vi "FGV_Instrument_Class.vi"(0 "Action":T2(ring), 5 "Instruments":T1(array[cluster]), 7 "Instr class":string, 9 "Instr name":string, 11 "error in (no error)":errorcluster, 12 "Parameter":string, 13 "Familly class IN":refnum<class "Class Instrument (Default).lvclass">) -> (4 "Instruments 2":T1(array[cluster]), 6 "Familly class Out":refnum<class "Class Instrument (Default).lvclass">, 15 "error out":errorcluster)   [LabVIEW 2020, in "Library Commun.lvlib"]
uses:
  Library Commun.lvlib
  Class/Instrument/Instrument (Default)/Class Instrument (Default).lvclass
  Class/Instrument/Instrument Firebase Altyor/Class Instrument Firebase Altyor.lvclass
  C:/Users/ngarcin/OneDrive - Altyor/Standard TB/Class/Instrument/Instrument (Default)/Class Instrument (Default).lvclass
  Class/Firebase/Source/Firebase Altyor/Firebase Altyor.lvclass
  Class/DIO/Class DIO NI/Class DIO NI.lvclass
  C:/Users/ngarcin/OneDrive - Altyor/Standard TB/Class/DIO/Class DIO (Default)/Class DIO (Default).lvclass
  TypeDef/Commande DIO/Parameter DIO.ctl
  Class/DIO/Class DIO (Default)/Class DIO (Default).lvclass
  Class/Instrument/Instrument DIO/Class Instrument DIO.lvclass
  Class/Ana/Class Ana NI/Class Ana NI.lvclass
  C:/Users/ngarcin/OneDrive - Altyor/Standard TB/Class/Ana/Class Ana (Default)/Class Ana (Default).lvclass
  Class/Ana/Class Ana (Default)/Class Ana (Default).lvclass
  Class/Instrument/Instrument Ana/Class Instrument Ana.lvclass
  Class/Multimeter/Multimeter Rigol DM3058/Class Multimeter Rigol DM3058.lvclass
  C:/Users/ngarcin/OneDrive - Altyor/Standard TB/Class/Multimeter/Multimeter (Default)/Class Multimeter (Default).lvclass
  Class/Multimeter/Multimeter (Default)/Class Multimeter (Default).lvclass
  TypeDef/Command Multimeter/Parameter Multimeter.ctl
  TypeDef/Command Multimeter/Typedef Function.ctl
  Class/Instrument/Class Instrument Multimeter/Class Instrument Multimeter.lvclass
  Class/Power_Supply/Power_Supply Rigol DP832/Class Power_Supply Rigol DP800.lvclass
  C:/Users/ngarcin/OneDrive - Altyor/Standard TB/Class/Power_Supply/Power_Supply (Default)/Power_Supply (Default).lvclass
  Class/Instrument/Instrument Power_Supply/Class Instrument Power_Supply.lvclass
  Class/Power_Supply/Power_Supply (Default)/Power_Supply (Default).lvclass
  TypeDef/Command Power_Supply/Parameter Power_Supply.ctl
  Class/Relay_Board/Relay_Board 16_Relay_Acer_Micro/Class Relay_Board 16_Relay_Acer_Micro.lvclass
  Class/Relay_Board/Relay_Board (Default)/Class Relay_Board (Default).lvclass
  Class/Instrument/Instrument Relay_Board/Class Instrument Relay_Board.lvclass
  Class/Relay_Board/Class Relay_Board 16_Relay_R4D3B16/Class Relay_Board 16_Relay_R4D3B16.lvclass
  C:/Users/ngarcin/OneDrive - Altyor/Standard TB/Class/Relay_Board/Relay_Board (Default)/Class Relay_Board (Default).lvclass
  TypeDef/Commande Relay_Board/Parameter Relay_Board.ctl
  Class/Relay_Board/Class Relay_Board 8_Relay_N4D8B08/Class Relay_Board 8_Relay_N4D8B08.lvclass
  Class/Relay_Board/Class Relay_Board 8_Relay_RY408D/Class Relay_Board 8_Relay_RY408D.lvclass
  Class/Relay_Board/Relay_Board usb_Relay_device/Class Relay_Board usb_Relay_device.lvclass
  TypeDef/Commande Printer/Commande Parameter Printer.ctl
  Class/Printer/Printer (Default)/Class Printer (Default).lvclass
  Class/Instrument/Instrument Printer/Class Instrument Printer.lvclass
  Class/Printer/Printer CAB/Class Printer_CAB.lvclass
  C:/Users/ngarcin/OneDrive - Altyor/Standard TB/Class/Printer/Printer (Default)/Class Printer (Default).lvclass
  Class/Printer/Printer TSC/Class Printer_TSC.lvclass
  Class/Instrument/Instrument Schielding_Box/Class Instrument Schielding_Box.lvclass
  Class/Shielding box/Class Shielding_ Box JC-PB3044/Class Shielding_ Box JC-PB3044.lvclass
  C:/Users/ngarcin/OneDrive - Altyor/Standard TB/Class/Shielding box/Class Shielding box (Default)/Class Shielding_ Box (Default).lvclass
  Class/Shielding box/Class Shielding box (Default)/Class Shielding_ Box (Default).lvclass
  TypeDef/Commande Shielding box/Commande Shielding box.ctl
  Class/Spectrum Analyser/Class Spectrum_Analyser RS306B/Class Spectrum_Analyser RS306B.lvclass
  C:/Users/ngarcin/OneDrive - Altyor/Standard TB/Class/Spectrum Analyser/Class Spectrum Analyser (Default)/Class Spectrum Analyser (Default).lvclass
  Class/Spectrum Analyser/Class Spectrum Analyser (Default)/Class Spectrum Analyser (Default).lvclass
  TypeDef/Command Spectrum_Analyser/Parameter Spectrum_Analyser.ctl
  Class/Instrument/Instrument Spectrum_Analyser/Class Instrument Spectrum_Analyser.lvclass
  TypeDef/Commande Led_Analyser/Parametre LED analyser.ctl
  Class/LED Analyser/Class Led Analyser (Default)/Class LED Analyser (Default).lvclass
  Class/LED Analyser/FEASA/LED Analyser FEASA_10_F/Class LED Analyser FEASA_10_F.lvclass
  C:/Users/ngarcin/OneDrive - Altyor/Standard TB/Class/LED Analyser/Class Led Analyser (Default)/Class LED Analyser (Default).lvclass
  Class/Instrument/Instrument LED_Analyser/Class Instrument LED_Analyser.lvclass
  TypeDef/Command firebase altyor/Parameter Firebase Altyor.ctl
  TypeDef/Bench Type.ctl
  Class/Firebase/Source/Firebase AssembledProducts/Firebase AssembledProducts.lvclass
  C:/Users/ngarcin/OneDrive - Altyor/Standard TB/Class/Firebase/Source/Firebase Altyor/Firebase Altyor.lvclass
  Class/Instrument/Instrument Database Altyor/Class Instrument Database Altyor.lvclass
  Class/Database/Database Altyor/Database Altyor.lvclass
  Class/Firebase/Source/Firebase PCBA/Firebase Benches.lvclass
  Class/Instrument/Instrument UART/Class Instrument UART.lvclass
  Class/UART/UART Enocean/Class UART Enocean.lvclass
  C:/Users/ngarcin/OneDrive - Altyor/Standard TB/Class/UART/UART (Default)/Class UART (Default).lvclass
  TypeDef/Commande UART/Parametre UART.ctl
  Class/UART/UART (Default)/Class UART (Default).lvclass
  Class/UART/UART Nodon/Class UART Nodon.lvclass
  Class/UART/UART P2056/Class UART P2056/Class UART P2056.lvclass
  Class/UART/UART Zigbee/Class UART Zigbee.lvclass
  Class/Camera/Class Camera IV3-500CA (Default)/Class Camera IV3-500CA.lvclass
  C:/Users/ngarcin/OneDrive - Altyor/Standard TB/Class/Camera/Class Camera Pattern Matching (Default)/Class Pattern Matching (Default).lvclass
  Class/Instrument/Instrument Pattern_Matching/Class Instrument Patterm_Matching.lvclass
  TypeDef/Commande Pattern_Matching/Commande Parameter.ctl
  Class/Camera/Class Camera Pattern Matching (Default)/Class Pattern Matching (Default).lvclass
  Class/Balance/Adam_GBK/Class Balance_Adam_GBK.lvclass
  C:/Users/ngarcin/OneDrive - Altyor/Standard TB/Class/Balance/Balance (Default)/Class Balance (Default).lvclass
  Class/Balance/Balance (Default)/Class Balance (Default).lvclass
  TypeDef/Commande Balance/Parameter Balance.ctl
  Class/Instrument/Instrument Balance/Class Instrument Balance.lvclass
  Class/Instrument/Instrument Log_File/Class Instrument Log_File.lvclass
  TypeDef/Commande Test/Commande Data Test.ctl
  TypeDef/Commande Test/Commande Value Type.ctl
  TypeDef/Commande Test/Commande Type Test.ctl
  Class/Log File/Class Log_File Altyor/Class Log_File Altyor.lvclass
  Class/JSON API/JSON Value/Set from JSON string.vi
  Class/JSON API/Variant JSON/Variant to JSON.vi
  Class/JSON API/JSON Value/Get Item by name array.vi
  Class/JSON API/JSON Value/JSON Value.lvclass
  Class/JSON API/Get Polymorphic/JSON GetSet.lvlib
  Class/JSON API/Variant JSON/Variant JSON.lvlib
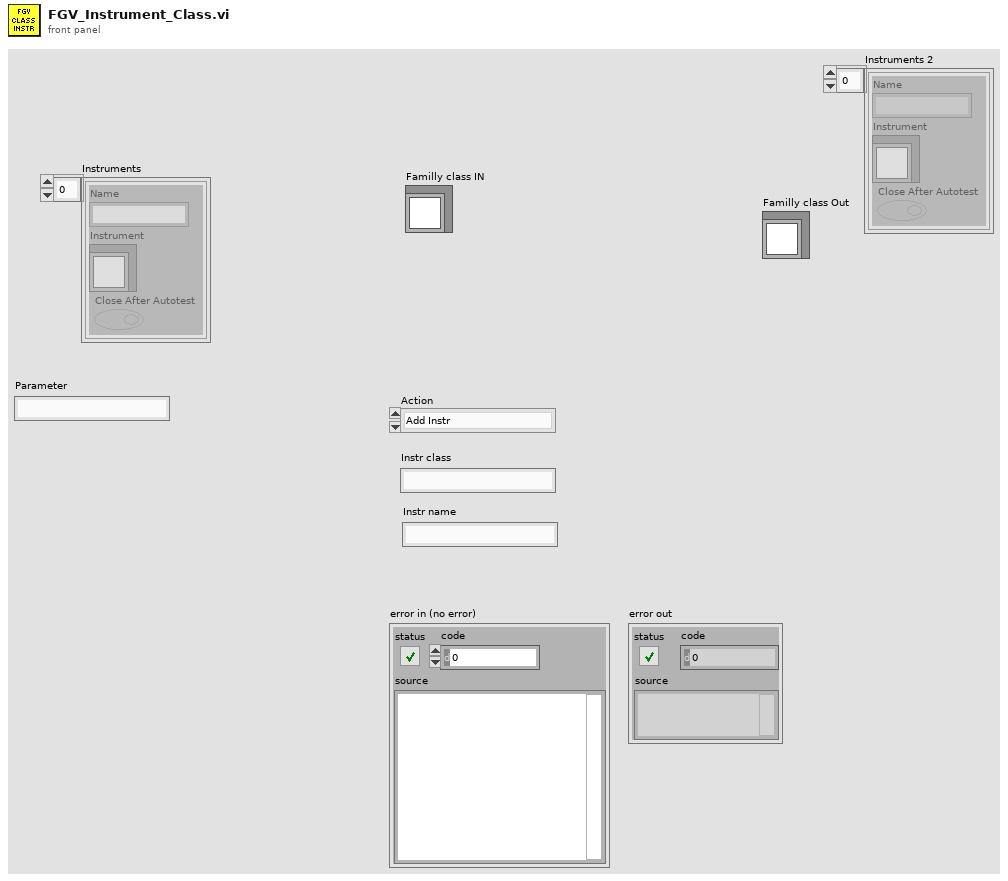
[diagram p1: front panel]
types:
  T1 = cluster{"Name":string, "Instrument":refnum<class "Class Instrument (Default).lvclass">, "Close After Autotest":bool}[]
  T2 = enum16{"Add Instr", "Remove Instr", "List Instr", "Get Instr Class", "Get Instr obj", "Save Insrt obj", "Modify Insrt obj", "Init"}
  T3 = typedef "Parameter DIO.ctl" = cluster{"Device_Com_Port":string, "Port":u8, "Line":u8, "Function":enum16{"Write", "Read"}, "Class DIO":refnum<class "Class DIO (Default).lvclass">}
  T4 = cluster{"Device_Com_Port":string, "Rate":u16, "Nb Sample":u16, "Voltage Max":dbl, "Voltage Min":dbl, "Input terminal Configuration":string, "Channel":u8[], "Continuous":bool, "Nb Data_To_Read":i16, "Class Ana":refnum<class "Class Ana (Default).lvclass">}
  T5 = typedef "Library Commun.lvlib/Parameter Multimeter.ctl" = cluster{"Device @":refnum<visa-resource-name>, "Range":dbl, "Voltage Type":enum16{"AC", "DC"}, "Function":T6, "Class Multimeter":refnum<class "Class Multimeter (Default).lvclass">}
  T6 = typedef "Library Commun.lvlib/Typedef Function.ctl" = enum16{"Voltmeter", "Ammeter", "Continuity", "Ohmmeter", "Frequencymeter"}
  T7 = typedef "Library Commun.lvlib/Parameter Relay_Board.ctl" = cluster{"Device_Com_Port":string, "Address Board":string, "Tab_Num_Relay":u8[], "Parameter Class Relay_Board":refnum<class "Class Relay_Board (Default).lvclass">}
  T8 = typedef "Commande Parameter Printer.ctl" = cluster{"Device_Printer":string, "File To print":path, "Path Picture":path, "Library Printer":refnum<class "Class Printer (Default).lvclass">}
  T9 = typedef "Commande Shielding box.ctl" = cluster{"Device @":string, "Class Shielding_ Box":refnum<class "Class Shielding_ Box (Default).lvclass">}
  T10 = typedef "Parameter Spectrum_Analyser.ctl" = cluster{"Device @":string, "Class Spectrum Analyser":refnum<class "Class Spectrum Analyser (Default).lvclass">, "Center Freq (MHz)":dbl, "Freq Span (MHz)":dbl, "Ref Level (dBm)":dbl, "Threshold (dBm)":dbl, "TimeOut":i16}
  T11 = typedef "Parametre LED analyser.ctl" = cluster{"Device @":string, "Channel":u16, "LED Analyser":refnum<class "Class LED Analyser (Default).lvclass">}
  T12 = typedef "Library Commun.lvlib/Parameter Firebase Altyor.ctl" = cluster{"Name_BDD":string, "API_Key":string, "Nb_to_Read":string, "Value_to_find":string, "Field_Filter":string, "Field_Order":string, "Collection_to_find":string, "Name_Bench":string, "Bench Type":T13, "Type Data ":enum16{"Data Product", "Data Test"}, "Firebase Altyor":refnum<class "Firebase Altyor.lvclass">}
  T13 = typedef "Library Commun.lvlib/Bench Type.ctl" = enum16{"Bench PCBA", "Bench Camera", "Bench Assembly", "Bench PCBA P2193"}
  T14 = cluster{"Connection Name ODBC":string, "DatabaseName":string, "Condition":string, "Type Data ":enum16{"Data Product", "Data Test"}, "Database Altyor":refnum<class "Database Altyor.lvclass">}
  T15 = typedef "Parametre UART.ctl" = cluster{"Address Device":refnum<visa-resource-name>, "Baud Rate":u32, "Data Bit":u16, "stop bits (10: 1 bit)":u16, "parity (0:none)":enum16{"None", "Odd", "Even", "Mark", "Space"}, "flow control (0:none)":u16, "termination char ":u8, "Enable Termination":bool, "Nb Octet to Read":u16, "Class UART":refnum<class "Class UART (Default).lvclass">}
  T16 = typedef "Commande Parameter.ctl" = cluster{"Device_Addr":string, "Port":string, "Number Prog":string, "Test Number":u16, "Timeout":u16, "Library Pattern Matching":refnum<class "Class Pattern Matching (Default).lvclass">}
  T17 = typedef "Parameter Balance.ctl" = cluster{"Device @":string, "Timeout":u32, "Class Balance":refnum<class "Class Balance (Default).lvclass">}
  T18 = cluster{"Path_Log_File":path, "Delimit":string, "File For Save":refnum<queue>, "Event Error":refnum<user-event>, "Class Log_File":refnum<class "Class Log_File Altyor.lvclass">}
  T19 = typedef "Library Commun.lvlib/Parameter Power_Supply.ctl" = cluster{"Device_Addr":refnum<visa-resource-name>, "Current":dbl, "Channel":i32, "Voltage":dbl, " Class Power_Supply":refnum<class "Power_Supply (Default).lvclass">}
  T20 = cluster{"Device_Com_Port":string, "Address Board":string}
  T21 = cluster{"Name_BDD":string, "API_Key":string, "Bench Type":T13}
  T22 = cluster{"Connection Name ODBC":string, "DatabaseName":string}
  T23 = cluster{"Address Device":refnum<visa-resource-name>, "Baud Rate":u32, "Data Bit":u16, "stop bits (10: 1 bit)":u16, "parity (0:none)":enum16{"None", "Odd", "Even", "Mark", "Space"}, "flow control (0:none)":u16, "termination char ":u8, "Enable Termination":bool}
  T24 = cluster{"Name":string, "Instrument":refnum<class "Class Instrument (Default).lvclass">, "Close After Autotest":bool}
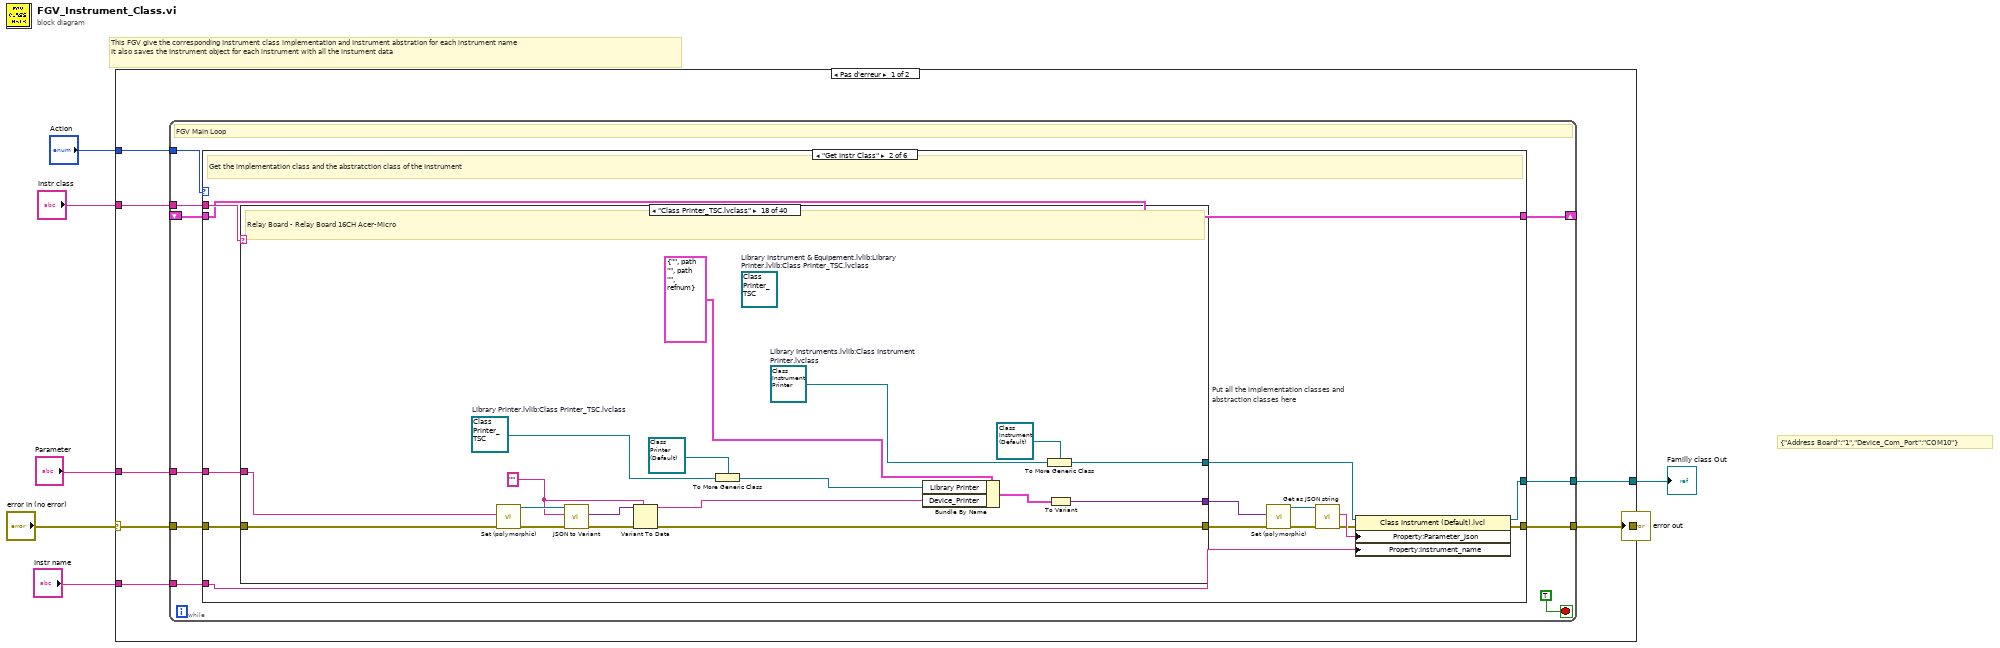
[diagram p0: block diagram]
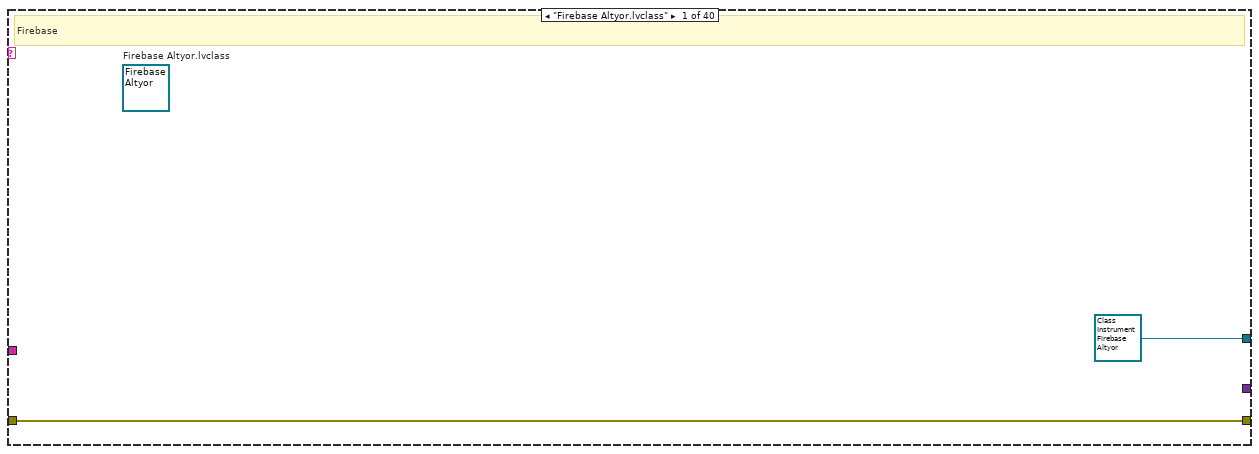
[diagram p3: hidden frame]
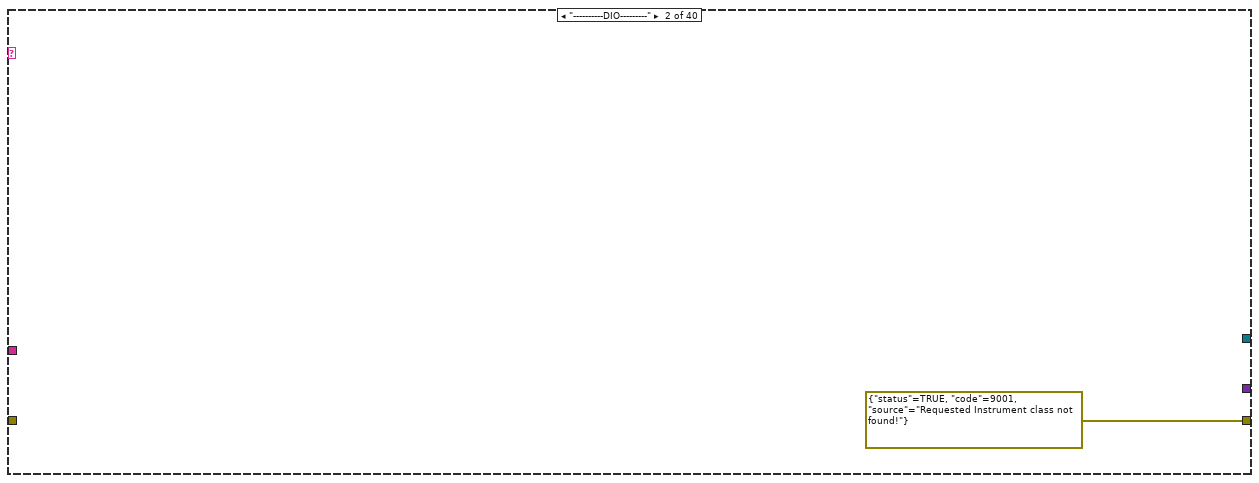
[diagram p4: hidden frame]
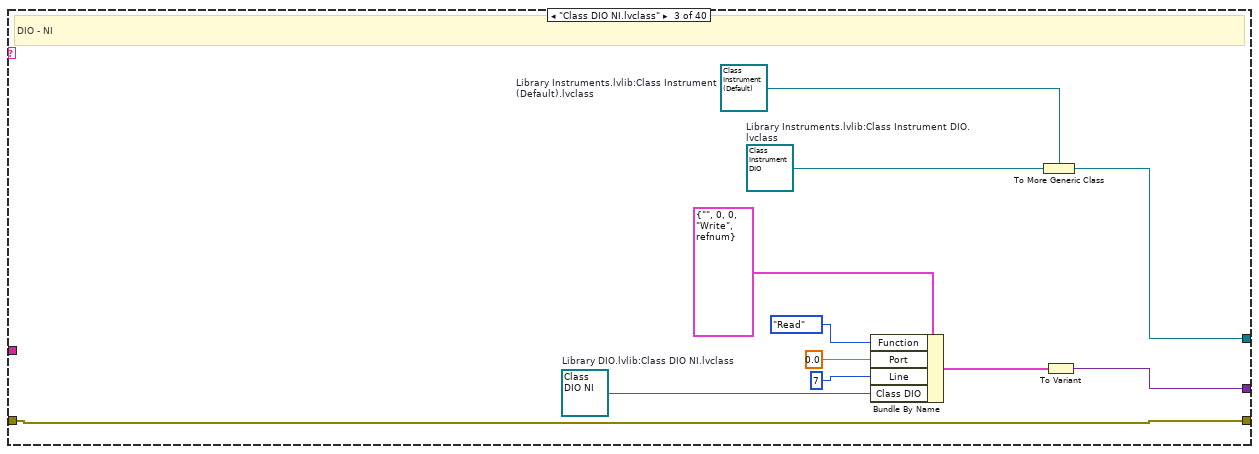
[diagram p5: hidden frame]
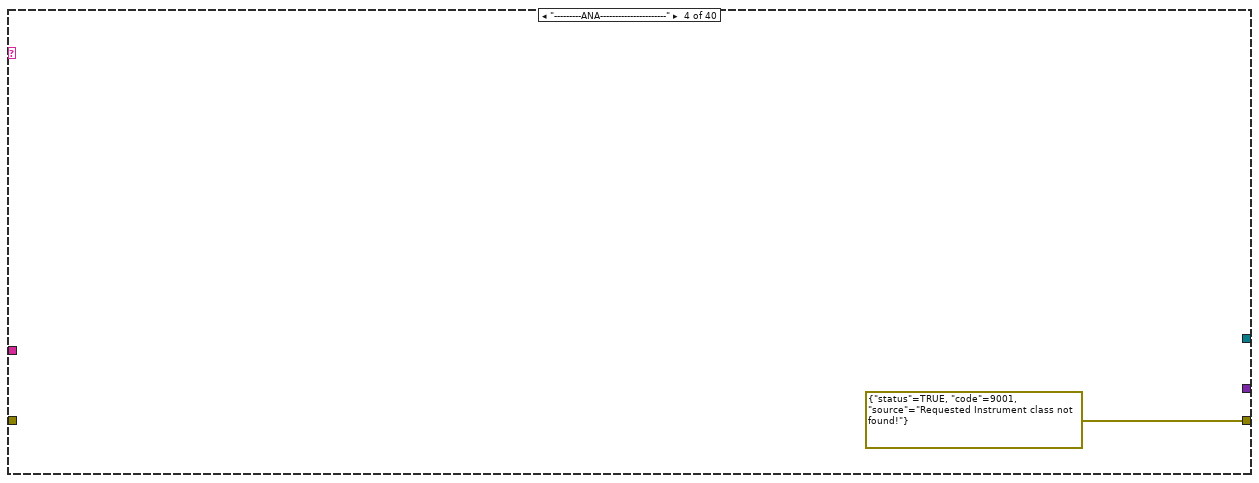
[diagram p6: hidden frame]
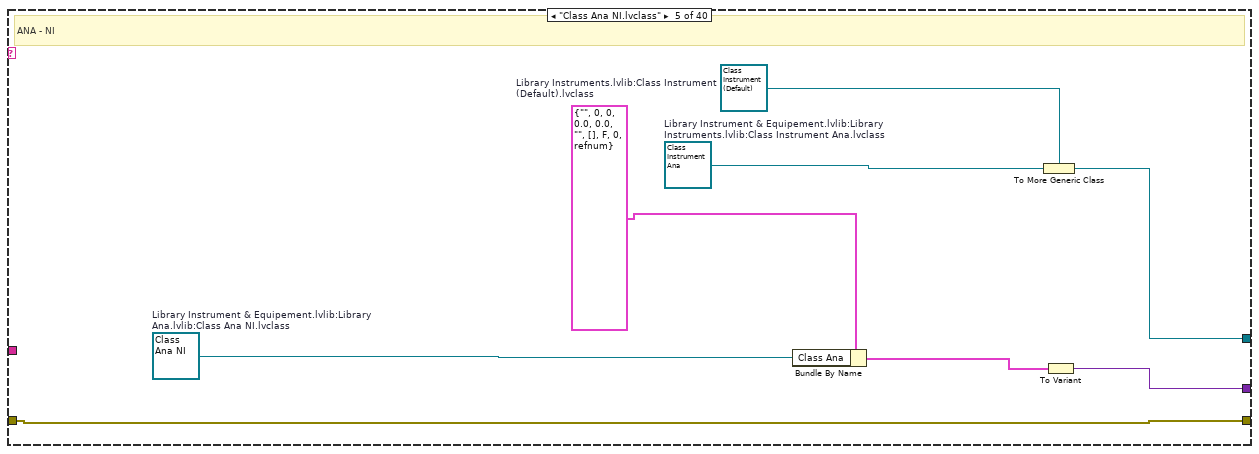
[diagram p7: hidden frame]
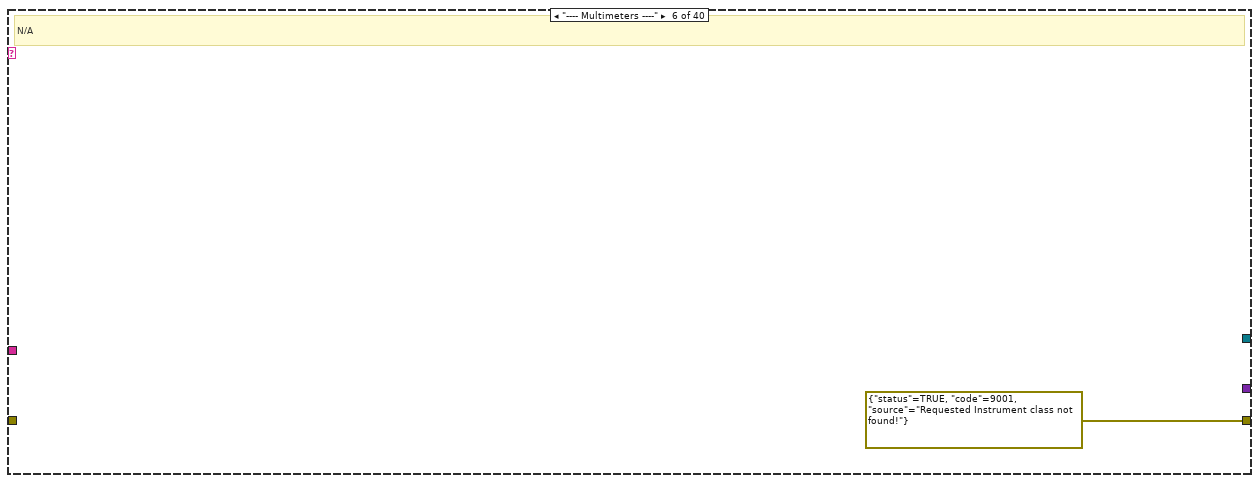
[diagram p8: hidden frame]
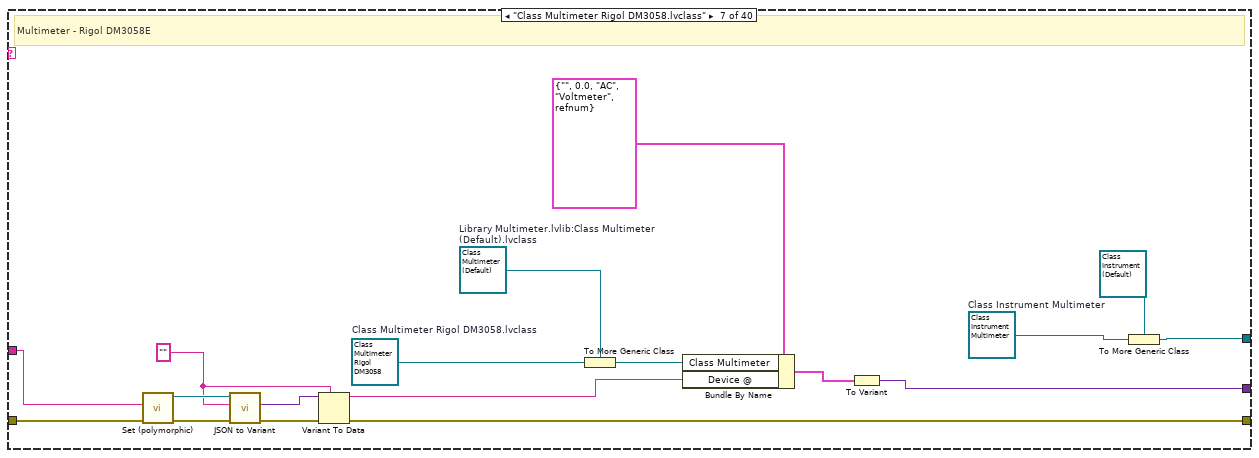
[diagram p9: hidden frame]
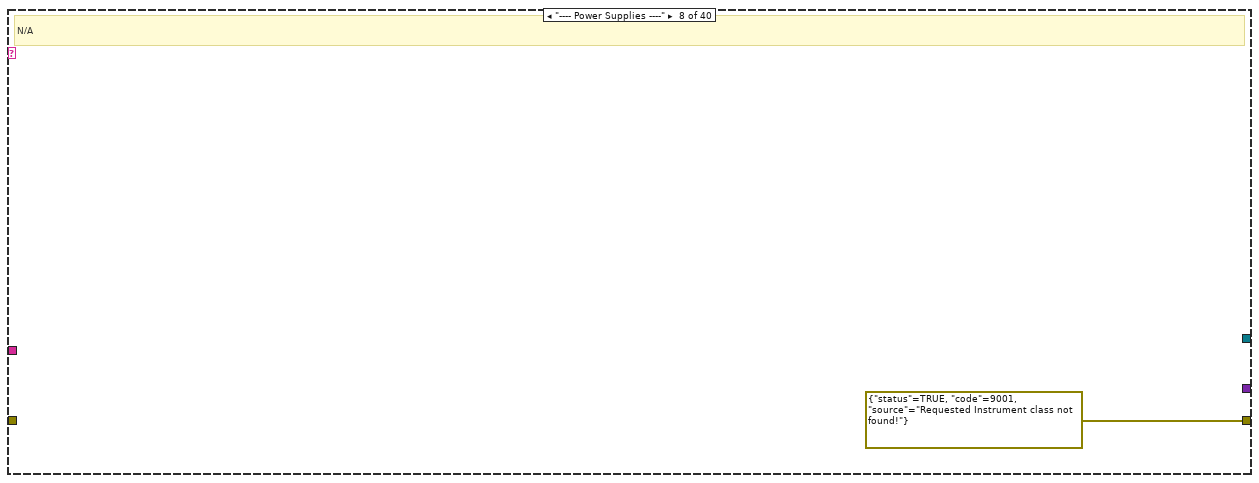
[diagram p10: hidden frame]
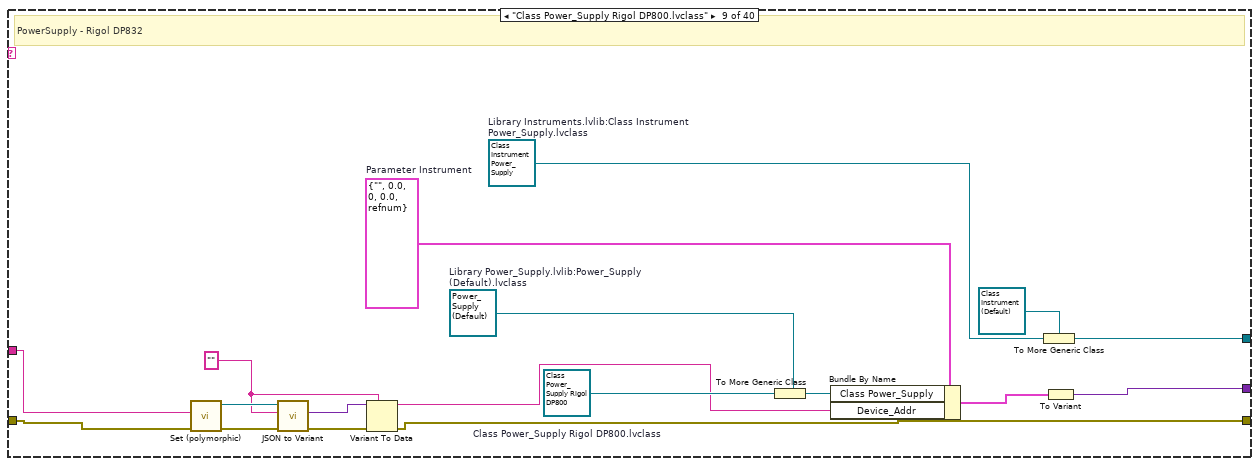
[diagram p11: hidden frame]
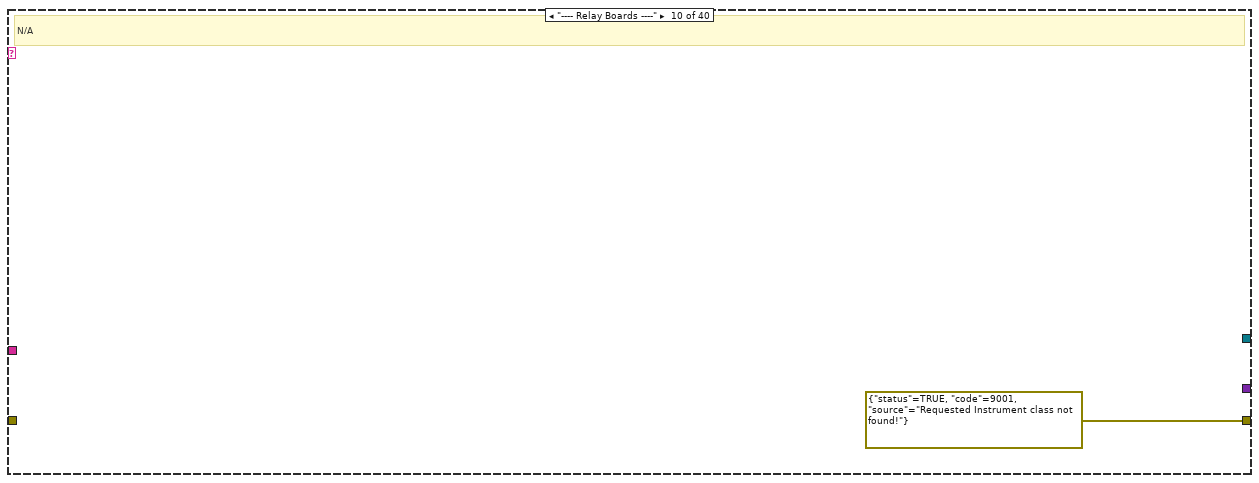
[diagram p12: hidden frame]
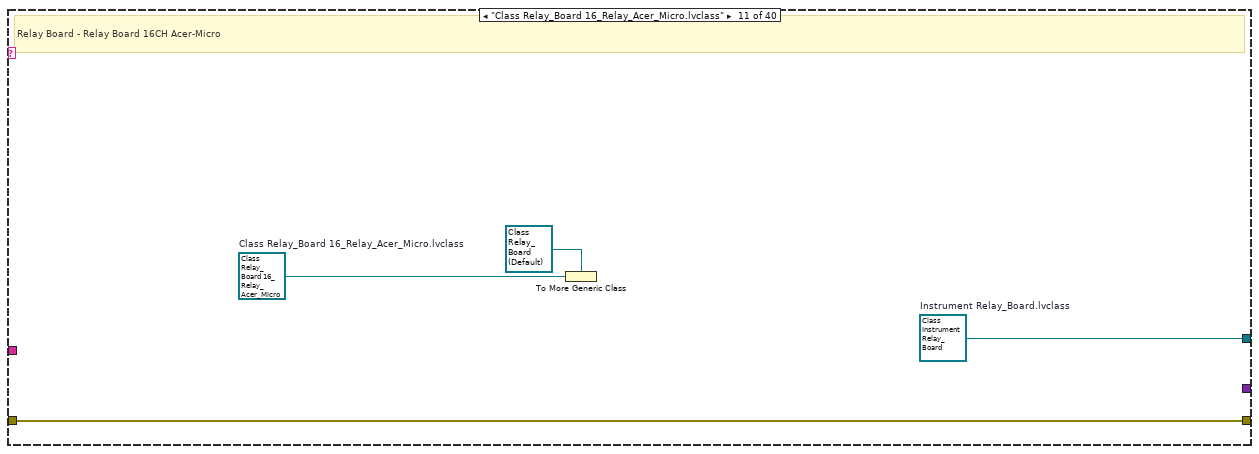
[diagram p13: hidden frame]
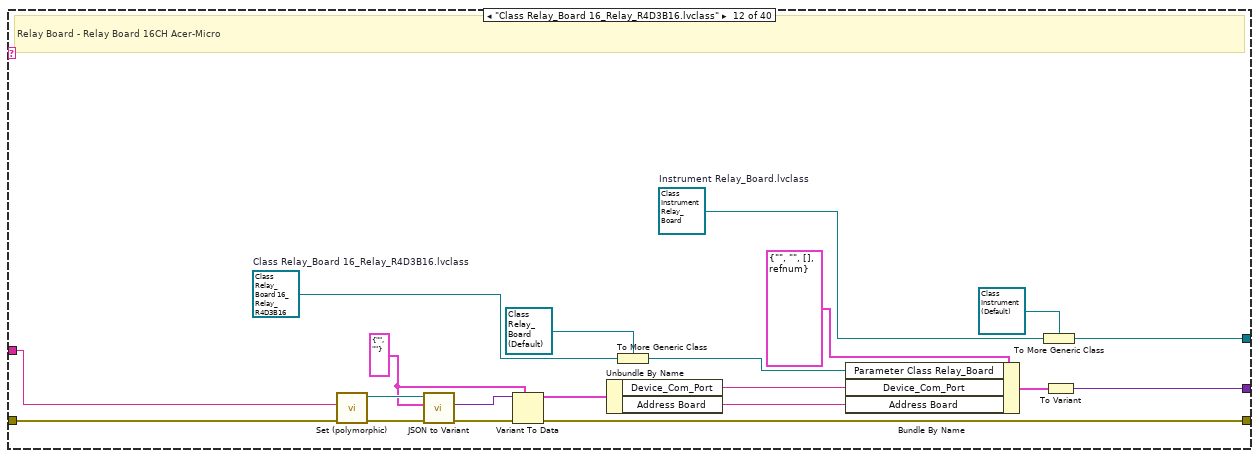
[diagram p14: hidden frame]
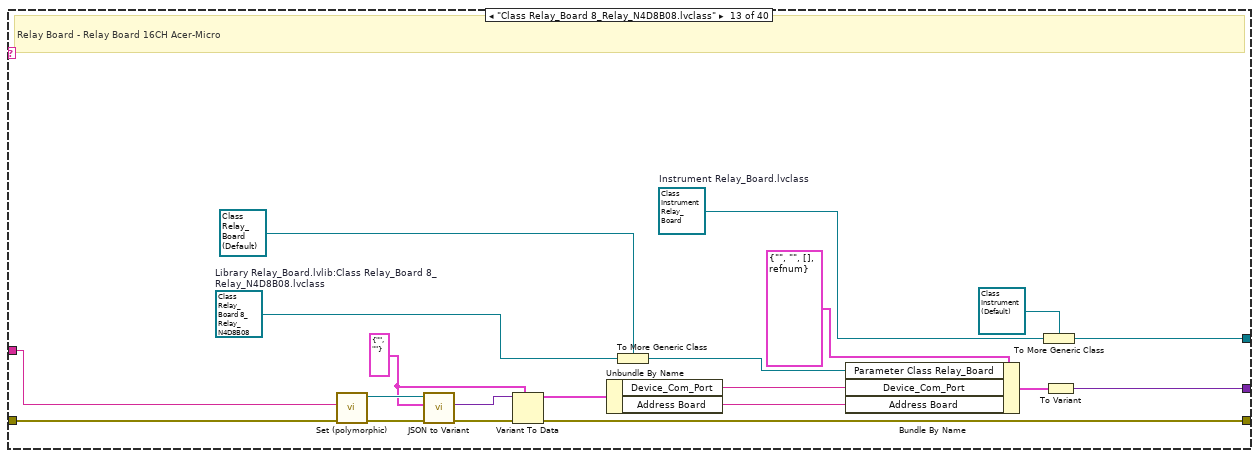
[diagram p15: hidden frame]
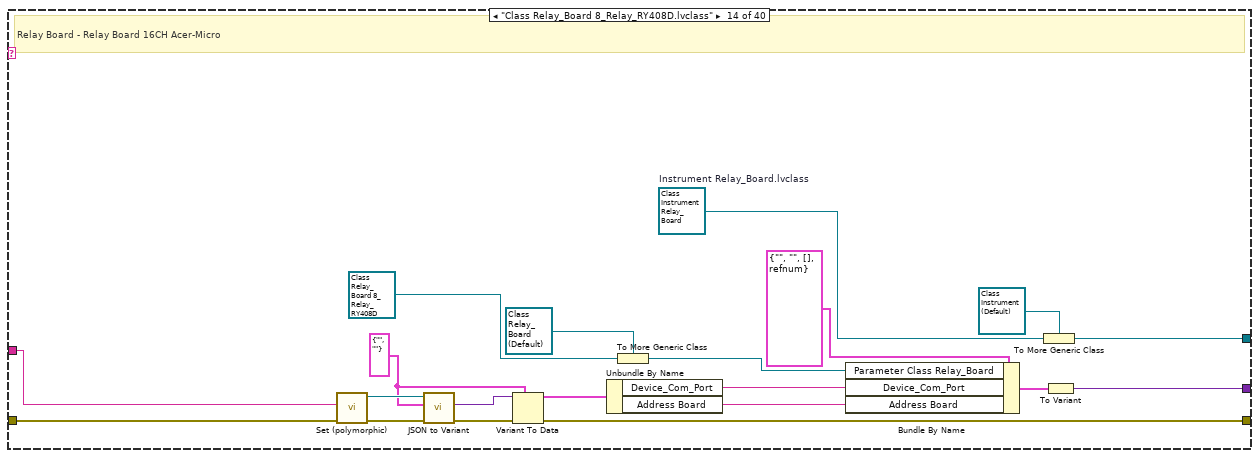
[diagram p16: hidden frame]
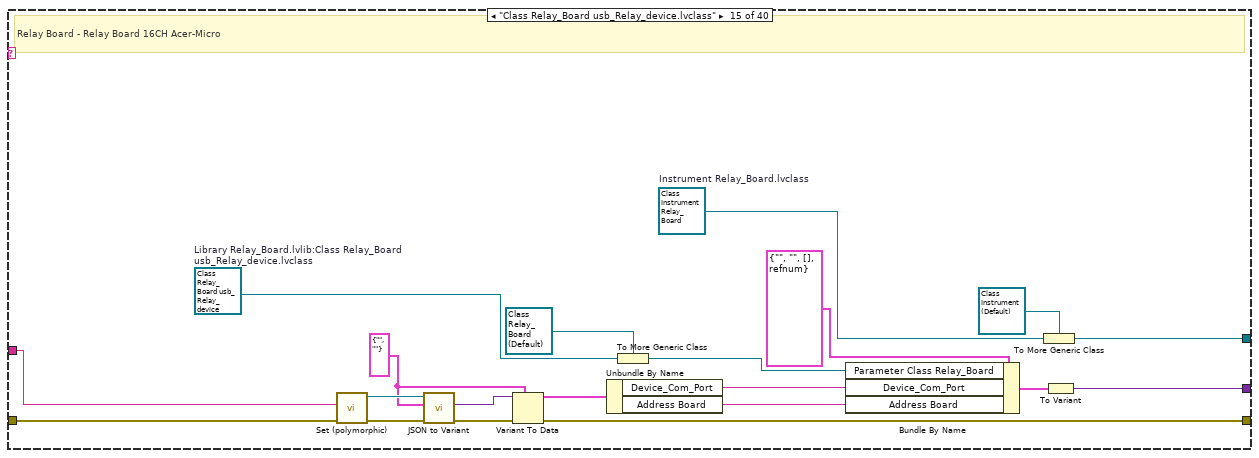
[diagram p17: hidden frame]
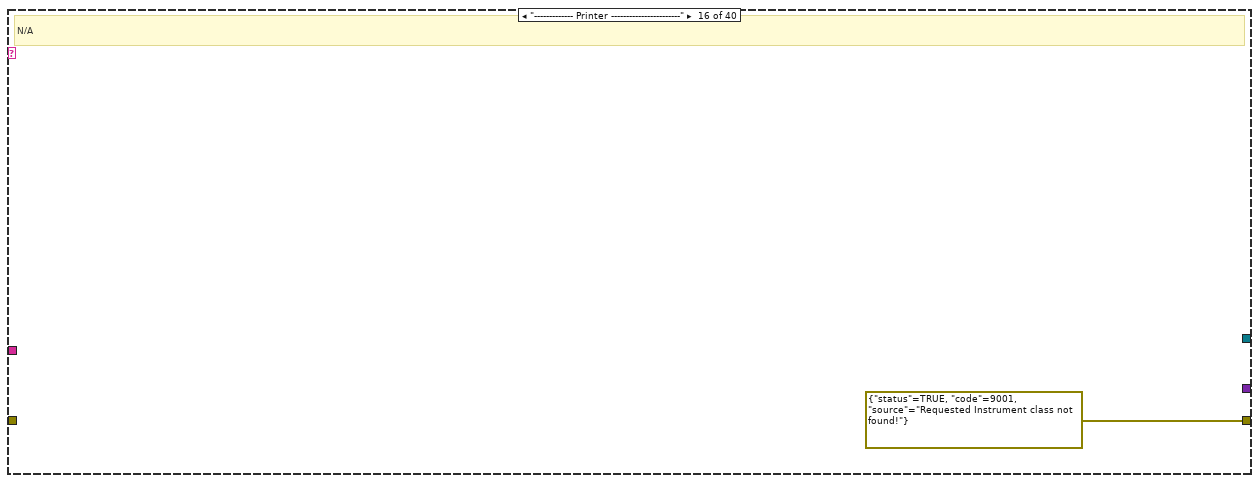
[diagram p18: hidden frame]
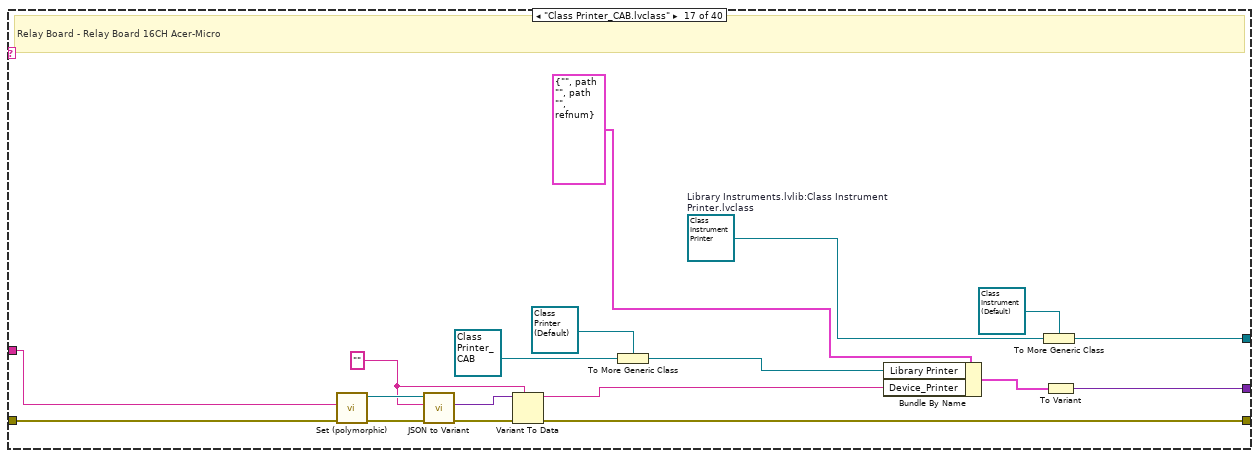
[diagram p19: hidden frame]
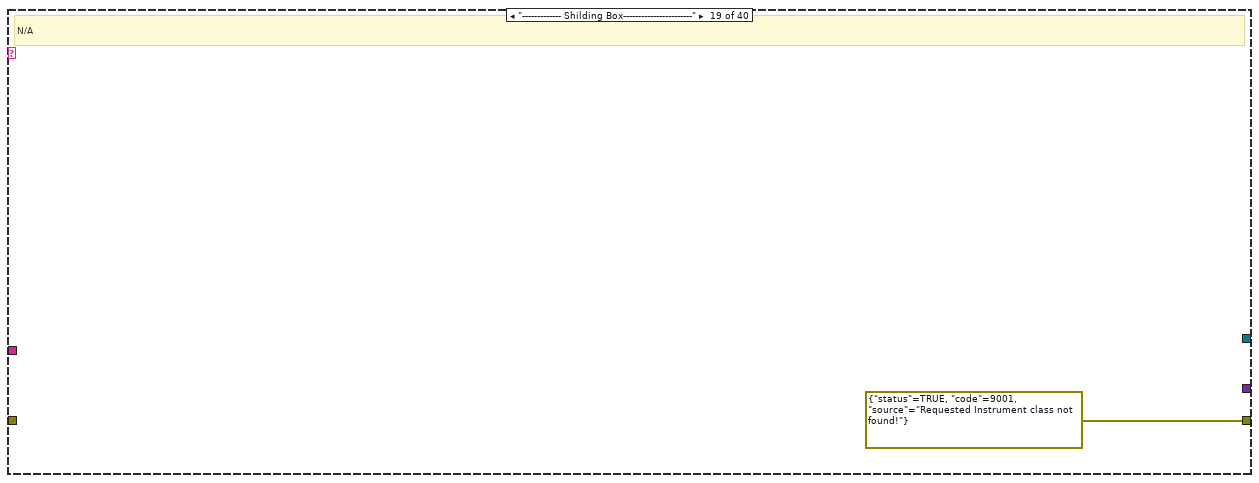
[diagram p20: hidden frame]
diagram:
  # "{\"Address Board\":\"1\",\"Device_Com_Port\":\"COM10\"}"
  # "This FGV give the corresponding Instrument class implementation and Instrument abstration for each instrument name\nIt also saves the Instrument object for each instrument with all the instument data"
  n1 = case shown="Pas d'erreur" "error in (no error)" {
    selector: "error in (no error)" -> [w13 w534]
    tunnel: [w12 w534] -> w6
    tunnel: "Action" -> [w14 _]
    tunnel: "Instr class" -> [w11 _]
    tunnel: "Instr name" -> [w10 _]
    tunnel: [w9 _] -> w2
    tunnel: "Parameter" -> [w8 _]
    frame No Error {
      n2 = while {
        tunnel: w14 -> [w24]
        tunnel: w13 -> [w23]
        tunnel: [w22] -> w12
        tunnel: w11 -> [w21]
        shift-right: [w17] -> _
        shift-left: _ -> [w20]
        tunnel: w10 -> [w18]
        tunnel: [w16] -> w9
        tunnel: w8 -> [w15]
        stop <- TRUE stop-if-true
        # "FGV Main Loop"
        n3 = case shown="\"Get Instr Class\"" w24 {
          tunnel: w23 -> [w26 w38 w500 w502 w518 w533]
          tunnel: [w26 w28 w500 w502 w518 w533] -> w22
          tunnel: w21 -> [_ w40 _ _ _ _]
          tunnel: w20 -> [w25 w39 _ w505 w516 w532]
          tunnel: w18 -> [_ w31 _ w504 w520 _]
          tunnel: [w25 w39 "Instruments" w505 w511 w532] -> w17
          tunnel: [_ w34 _ w503 w519 _] -> w16
          tunnel: w15 -> [_ w30 _ _ _ _]
          frame "Init", Default {
            # "Init the FGV"
          }
          frame "Get Instr Class" {
            # "Get the implementation class and the abstratction class of the Instrument"
            n4 = case "Put all the implementation classes and abstraction classes here" shown="\"Class Printer_TSC.lvclass\"" w40 {
              tunnel: w38 -> [w42 _ w54 _ w63 _ w71 _ w86 _ w106 w116 w137 w157 w177 _ w198 w216 _ w235 _ w252 _ w271 _ w293 w312 w332 _ w360 w384 w408 w432 _ w452 _ w472 _ w492 _]
              tunnel: [w42 errorcluster {"status"=TRUE, "code"=9001, "source"="Requested Instrument class not found!"} ("error constant") w54 errorcluster {"status"=TRUE, "code"=9001, "source"="Requested Instrument class not found!"} ("error constant") w63 errorcluster {"status"=TRUE, "code"=9001, "source"="Requested Instrument class not found!"} ("error constant") w70 errorcluster {"status"=TRUE, "code"=9001, "source"="Requested Instrument class not found!"} ("error constant") w85 errorcluster {"status"=TRUE, "code"=9001, "source"="Requested Instrument class not found!"} ("error constant") w106 w107 w128 w148 w168 errorcluster {"status"=TRUE, "code"=9001, "source"="Requested Instrument class not found!"} ("error constant") w194 w212 errorcluster {"status"=TRUE, "code"=9001, "source"="Requested Instrument class not found!"} ("error constant") w231 errorcluster {"status"=TRUE, "code"=9001, "source"="Requested Instrument class not found!"} ("error constant") w251 errorcluster {"status"=TRUE, "code"=9001, "source"="Requested Instrument class not found!"} ("error constant") w270 errorcluster {"status"=TRUE, "code"=9001, "source"="Requested Instrument class not found!"} ("error constant") w285 w305 w324 errorcluster {"status"=TRUE, "code"=9001, "source"="Requested Instrument class not found!"} ("error constant") w356 w380 w404 w428 errorcluster {"status"=TRUE, "code"=9001, "source"="Requested Instrument class not found!"} ("error constant") w448 errorcluster {"status"=TRUE, "code"=9001, "source"="Requested Instrument class not found!"} ("error constant") w471 errorcluster {"status"=TRUE, "code"=9001, "source"="Requested Instrument class not found!"} ("error constant") w489 errorcluster {"status"=TRUE, "code"=9001, "source"="Requested Instrument class not found!"} ("error constant")] -> w36
              tunnel: [refnum<class "Class Instrument Firebase Altyor.lvclass"> refnum ("Library Instruments.lvlib:Class Instrument Firebase Altyor.lvclass") _ w52 _ w61 _ w66 _ w95 _ w103 w122 w143 w163 w183 _ w204 w222 _ w241 _ w248 _ w267 _ w299 w317 w338 _ w365 w389 w413 w437 _ w457 _ w468 _ w497 _] -> w35
              tunnel: [_ _ w45 _ w59 _ w73 _ w97 _ _ w121 w142 w162 w182 _ w203 w221 _ w240 _ w254 _ w273 _ w289 w309 w329 _ w357 w381 w405 w429 _ w449 _ w474 _ w490 _] -> w27
              tunnel: w30 -> [_ _ _ _ _ _ w72 _ w87 _ _ w114 w135 w155 w175 _ w197 w215 _ w234 _ w253 _ w272 _ w292 w311 w319 _ w359 w383 w407 w431 _ w451 _ w473 _ w481 _]
              frame "Firebase Altyor.lvclass" {
                (unwired) refnum<class "Firebase Altyor.lvclass"> refnum  # Firebase Altyor.lvclass
                # "Firebase"
              }
              frame "----------DIO---------" {
              }
              frame "Class DIO NI.lvclass" {
                w44 = refnum<class "Class Instrument DIO.lvclass"> refnum  # Library Instruments.lvlib:Class Instrument DIO.lvclass
                w47 = refnum<class "Class DIO NI.lvclass"> refnum  # Library DIO.lvlib:Class DIO NI.lvclass
                w53 = refnum<class "Class Instrument (Default).lvclass"> refnum  # Library Instruments.lvlib:Class Instrument (Default).lvclass
                # "DIO - NI"
                n5 = Bundle By Name(cluster=T3 {"Device_Com_Port"="", "Port"=0, "Line"=0, "Function"=enum."Write", "Class DIO"=refnum} ("Parameter"), "Function"=enum16{"Write", "Read"}."Read", "Port"=0.0 ("Range"), "Line"=7 ("Channel"), "Class DIO"=w47) -> (w46:T3)
                n6 = To More Generic Class(target class=w53, reference=w44) -> (generic class reference=w52:refnum<class "Class Instrument (Default).lvclass">)
                n7 = To Variant(anything=w46) -> (Variant=w45:variant)
              }
              frame "---------ANA----------------------" {
              }
              frame "Class Ana NI.lvclass" {
                w56 = refnum<class "Class Instrument Ana.lvclass"> refnum  # Library Instrument & Equipement.lvlib:Library Instruments.lvlib:Class Instrument Ana.lvclass
                w57 = refnum<class "Class Ana NI.lvclass"> refnum  # Library Instrument & Equipement.lvlib:Library Ana.lvlib:Class Ana NI.lvclass
                w62 = refnum<class "Class Instrument (Default).lvclass"> refnum  # Library Instruments.lvlib:Class Instrument (Default).lvclass
                # "ANA - NI"
                n8 = Bundle By Name(cluster=T4 {"Device_Com_Port"="", "Rate"=0, "Nb Sample"=0, "Voltage Max"=0.0, "Voltage Min"=0.0, "Input terminal Configuration"="", "Channel"=[], "Continuous"=FALSE, "Nb Data_To_Read"=0, "Class Ana"=refnum} ("Parameter"), "Class Ana"=w57) -> (w60:T4)
                n9 = To More Generic Class(target class=w62, reference=w56) -> (generic class reference=w61:refnum<class "Class Instrument (Default).lvclass">)
                n10 = To Variant(anything=w60) -> (Variant=w59:variant)
              }
              frame "---- Multimeters ----" {
                # "N/A"
              }
              frame "Class Multimeter Rigol DM3058.lvclass" {
                w65 = refnum<class "Class Instrument Multimeter.lvclass"> refnum  # Class Instrument Multimeter
                w75 = "" ("Address Board")
                w81 = refnum<class "Class Multimeter (Default).lvclass"> refnum  # Library Multimeter.lvlib:Class Multimeter (Default).lvclass
                w82 = refnum<class "Class Multimeter Rigol DM3058.lvclass"> refnum  # Class Multimeter Rigol DM3058.lvclass
                # "Multimeter - Rigol DM3058E"
                n11 = call-poly "Set (polymorphic).vi"("error in (no error)"=w71, "JSON stream"=w72) -> ("error out"=w79:errorcluster, "JSON Value out"=w77:refnum<class "JSON Value.lvclass">)  [unwired: 7 in, 1 out]
                n12 = call "JSON to Variant.vi"("error in (no error)"=w79, "Variant (Data Type)"=w75, "JSON Value"=w77) -> ("error out"=w78:errorcluster, "Variant out"=w80:variant)  [unwired: 7 in]
                n13 = Variant To Data(error in=w78, type=w75, Variant=w80) -> (data=w74:string, error out=w70:errorcluster)
                n14 = To More Generic Class(target class=w81, reference=w82) -> (generic class reference=w68:refnum<class "Class Multimeter (Default).lvclass">)
                n15 = Bundle By Name(cluster=T5 {"Device @"="", "Range"=0.0, "Voltage Type"=enum."AC", "Function"=enum."Voltmeter", "Class Multimeter"=refnum} ("Parameter"), "Class Multimeter"=w68, "Device @"=w74) -> (w76:T5)
                n16 = To Variant(anything=w76) -> (Variant=w73:variant)
                n17 = To More Generic Class(target class=refnum<class "Class Instrument (Default).lvclass"> refnum ("Library Instruments.lvlib:Class Instrument (Default).lvclass"), reference=w65) -> (generic class reference=w66:refnum<class "Class Instrument (Default).lvclass">)
              }
              frame "---- Power Supplies ----" {
                # "N/A"
              }
              frame "Class Power_Supply Rigol DP800.lvclass" {
                w88 = "" ("Address Board")
                w93 = T19 {"Device_Addr"="", "Current"=0.0, "Channel"=0, "Voltage"=0.0, " Class Power_Supply"=refnum}  # Parameter Instrument
                w100 = refnum<class "Power_Supply (Default).lvclass"> refnum  # Library Power_Supply.lvlib:Power_Supply (Default).lvclass
                w96 = refnum<class "Class Instrument Power_Supply.lvclass"> refnum  # Library Instruments.lvlib:Class Instrument Power_Supply.lvclass
                w101 = refnum<class "Class Power_Supply Rigol DP800.lvclass"> refnum  # Class Power_Supply Rigol DP800.lvclass
                # "PowerSupply - Rigol DP832"
                n18 = call-poly "Set (polymorphic).vi"("error in (no error)"=w86, "JSON stream"=w87) -> ("error out"=w91:errorcluster, "JSON Value out"=w89:refnum<class "JSON Value.lvclass">)  [unwired: 7 in, 1 out]
                n19 = call "JSON to Variant.vi"("error in (no error)"=w91, "Variant (Data Type)"=w88, "JSON Value"=w89) -> ("error out"=w90:errorcluster, "Variant out"=w92:variant)  [unwired: 7 in]
                n20 = Variant To Data(error in=w90, type=w88, Variant=w92) -> (data=w84:string, error out=w85:errorcluster)
                n21 = To More Generic Class(target class=w100, reference=w101) -> (generic class reference=w99:refnum<class "Power_Supply (Default).lvclass">)
                n22 = Bundle By Name(cluster=w93, "Class Power_Supply"=w99, "Device_Addr"=w84) -> (w98:T19)
                n23 = To More Generic Class(target class=refnum<class "Class Instrument (Default).lvclass"> refnum ("Library Instruments.lvlib:Class Instrument (Default).lvclass"), reference=w96) -> (generic class reference=w95:refnum<class "Class Instrument (Default).lvclass">)
                n24 = To Variant(anything=w98) -> (Variant=w97:variant)
              }
              frame "---- Relay Boards ----" {
                # "N/A"
              }
              frame "Class Relay_Board 16_Relay_Acer_Micro.lvclass" {
                w103 = refnum<class "Class Instrument Relay_Board.lvclass"> refnum  # Instrument Relay_Board.lvclass
                w105 = refnum<class "Class Relay_Board 16_Relay_Acer_Micro.lvclass"> refnum  # Class Relay_Board 16_Relay_Acer_Micro.lvclass
                # "Relay Board - Relay Board 16CH Acer-Micro"
                n25 = To More Generic Class(target class=refnum<class "Class Relay_Board (Default).lvclass"> refnum ("Library Relay_Board.lvlib:Class Relay_Board (Default).lvclass"), reference=w105) -> ()  [unwired: 1 out]
              }
              frame "Class Relay_Board 16_Relay_R4D3B16.lvclass" {
                w115 = T20 {"Device_Com_Port"="", "Address Board"=""} ("Parameter")
                w123 = refnum<class "Class Instrument Relay_Board.lvclass"> refnum  # Instrument Relay_Board.lvclass
                w125 = refnum<class "Class Relay_Board 16_Relay_R4D3B16.lvclass"> refnum  # Class Relay_Board 16_Relay_R4D3B16.lvclass
                # "Relay Board - Relay Board 16CH Acer-Micro"
                n26 = call-poly "Set (polymorphic).vi"("error in (no error)"=w116, "JSON stream"=w114) -> ("error out"=w119:errorcluster, "JSON Value out"=w117:refnum<class "JSON Value.lvclass">)  [unwired: 7 in, 1 out]
                n27 = call "JSON to Variant.vi"("error in (no error)"=w119, "Variant (Data Type)"=w115, "JSON Value"=w117) -> ("error out"=w118:errorcluster, "Variant out"=w120:variant)  [unwired: 7 in]
                n28 = Variant To Data(error in=w118, type=w115, Variant=w120) -> (data=w112:T20, error out=w107:errorcluster)
                n29 = Unbundle By Name(w112) -> ("Device_Com_Port"=w111:string, "Address Board"=w110:string)
                n30 = To More Generic Class(target class=refnum<class "Class Relay_Board (Default).lvclass"> refnum ("Library Relay_Board.lvlib:Class Relay_Board (Default).lvclass"), reference=w125) -> (generic class reference=w109:refnum<class "Class Relay_Board (Default).lvclass">)
                n31 = Bundle By Name(cluster=T7 {"Device_Com_Port"="", "Address Board"="", "Tab_Num_Relay"=[], "Parameter Class Relay_Board"=refnum} ("Parameter"), "Parameter Class Relay_Board"=w109, "Device_Com_Port"=w111, "Address Board"=w110) -> (w108:T7)
                n32 = To More Generic Class(target class=refnum<class "Class Instrument (Default).lvclass"> refnum ("Library Instruments.lvlib:Class Instrument (Default).lvclass"), reference=w123) -> (generic class reference=w122:refnum<class "Class Instrument (Default).lvclass">)
                n33 = To Variant(anything=w108) -> (Variant=w121:variant)
              }
              frame "Class Relay_Board 8_Relay_N4D8B08.lvclass" {
                w127 = refnum<class "Class Relay_Board 8_Relay_N4D8B08.lvclass"> refnum  # Library Relay_Board.lvlib:Class Relay_Board 8_Relay_N4D8B08.lvclass
                w136 = T20 {"Device_Com_Port"="", "Address Board"=""} ("Parameter")
                w144 = refnum<class "Class Instrument Relay_Board.lvclass"> refnum  # Instrument Relay_Board.lvclass
                # "Relay Board - Relay Board 16CH Acer-Micro"
                n34 = call-poly "Set (polymorphic).vi"("error in (no error)"=w137, "JSON stream"=w135) -> ("error out"=w140:errorcluster, "JSON Value out"=w138:refnum<class "JSON Value.lvclass">)  [unwired: 7 in, 1 out]
                n35 = call "JSON to Variant.vi"("error in (no error)"=w140, "Variant (Data Type)"=w136, "JSON Value"=w138) -> ("error out"=w139:errorcluster, "Variant out"=w141:variant)  [unwired: 7 in]
                n36 = Variant To Data(error in=w139, type=w136, Variant=w141) -> (data=w133:T20, error out=w128:errorcluster)
                n37 = Unbundle By Name(w133) -> ("Device_Com_Port"=w132:string, "Address Board"=w131:string)
                n38 = To More Generic Class(target class=refnum<class "Class Relay_Board (Default).lvclass"> refnum ("Library Relay_Board.lvlib:Class Relay_Board (Default).lvclass"), reference=w127) -> (generic class reference=w130:refnum<class "Class Relay_Board (Default).lvclass">)
                n39 = Bundle By Name(cluster=T7 {"Device_Com_Port"="", "Address Board"="", "Tab_Num_Relay"=[], "Parameter Class Relay_Board"=refnum} ("Parameter"), "Parameter Class Relay_Board"=w130, "Device_Com_Port"=w132, "Address Board"=w131) -> (w129:T7)
                n40 = To More Generic Class(target class=refnum<class "Class Instrument (Default).lvclass"> refnum ("Library Instruments.lvlib:Class Instrument (Default).lvclass"), reference=w144) -> (generic class reference=w143:refnum<class "Class Instrument (Default).lvclass">)
                n41 = To Variant(anything=w129) -> (Variant=w142:variant)
              }
              frame "Class Relay_Board 8_Relay_RY408D.lvclass" {
                w156 = T20 {"Device_Com_Port"="", "Address Board"=""} ("Parameter")
                w164 = refnum<class "Class Instrument Relay_Board.lvclass"> refnum  # Instrument Relay_Board.lvclass
                # "Relay Board - Relay Board 16CH Acer-Micro"
                n42 = call-poly "Set (polymorphic).vi"("error in (no error)"=w157, "JSON stream"=w155) -> ("error out"=w160:errorcluster, "JSON Value out"=w158:refnum<class "JSON Value.lvclass">)  [unwired: 7 in, 1 out]
                n43 = call "JSON to Variant.vi"("error in (no error)"=w160, "Variant (Data Type)"=w156, "JSON Value"=w158) -> ("error out"=w159:errorcluster, "Variant out"=w161:variant)  [unwired: 7 in]
                n44 = Variant To Data(error in=w159, type=w156, Variant=w161) -> (data=w153:T20, error out=w148:errorcluster)
                n45 = Unbundle By Name(w153) -> ("Device_Com_Port"=w152:string, "Address Board"=w151:string)
                n46 = To More Generic Class(target class=refnum<class "Class Relay_Board (Default).lvclass"> refnum ("Library Relay_Board.lvlib:Class Relay_Board (Default).lvclass"), reference=refnum<class "Class Relay_Board 8_Relay_RY408D.lvclass"> refnum ("Library Relay_Board.lvlib:Class Relay_Board 8_Relay_RY408D.lvclass")) -> (generic class reference=w150:refnum<class "Class Relay_Board (Default).lvclass">)
                n47 = Bundle By Name(cluster=T7 {"Device_Com_Port"="", "Address Board"="", "Tab_Num_Relay"=[], "Parameter Class Relay_Board"=refnum} ("Parameter"), "Parameter Class Relay_Board"=w150, "Device_Com_Port"=w152, "Address Board"=w151) -> (w149:T7)
                n48 = To More Generic Class(target class=refnum<class "Class Instrument (Default).lvclass"> refnum ("Library Instruments.lvlib:Class Instrument (Default).lvclass"), reference=w164) -> (generic class reference=w163:refnum<class "Class Instrument (Default).lvclass">)
                n49 = To Variant(anything=w149) -> (Variant=w162:variant)
              }
              frame "Class Relay_Board usb_Relay_device.lvclass" {
                w167 = refnum<class "Class Relay_Board usb_Relay_device.lvclass"> refnum  # Library Relay_Board.lvlib:Class Relay_Board usb_Relay_device.lvclass
                w176 = T20 {"Device_Com_Port"="", "Address Board"=""} ("Parameter")
                w184 = refnum<class "Class Instrument Relay_Board.lvclass"> refnum  # Instrument Relay_Board.lvclass
                # "Relay Board - Relay Board 16CH Acer-Micro"
                n50 = call-poly "Set (polymorphic).vi"("error in (no error)"=w177, "JSON stream"=w175) -> ("error out"=w180:errorcluster, "JSON Value out"=w178:refnum<class "JSON Value.lvclass">)  [unwired: 7 in, 1 out]
                n51 = call "JSON to Variant.vi"("error in (no error)"=w180, "Variant (Data Type)"=w176, "JSON Value"=w178) -> ("error out"=w179:errorcluster, "Variant out"=w181:variant)  [unwired: 7 in]
                n52 = Variant To Data(error in=w179, type=w176, Variant=w181) -> (data=w173:T20, error out=w168:errorcluster)
                n53 = Unbundle By Name(w173) -> ("Device_Com_Port"=w172:string, "Address Board"=w171:string)
                n54 = To More Generic Class(target class=refnum<class "Class Relay_Board (Default).lvclass"> refnum ("Library Relay_Board.lvlib:Class Relay_Board (Default).lvclass"), reference=w167) -> (generic class reference=w170:refnum<class "Class Relay_Board (Default).lvclass">)
                n55 = Bundle By Name(cluster=T7 {"Device_Com_Port"="", "Address Board"="", "Tab_Num_Relay"=[], "Parameter Class Relay_Board"=refnum} ("Parameter"), "Parameter Class Relay_Board"=w170, "Device_Com_Port"=w172, "Address Board"=w171) -> (w169:T7)
                n56 = To More Generic Class(target class=refnum<class "Class Instrument (Default).lvclass"> refnum ("Library Instruments.lvlib:Class Instrument (Default).lvclass"), reference=w184) -> (generic class reference=w183:refnum<class "Class Instrument (Default).lvclass">)
                n57 = To Variant(anything=w169) -> (Variant=w182:variant)
              }
              frame "------------- Printer -----------------------" {
                # "N/A"
              }
              frame "Class Printer_CAB.lvclass" {
                w191 = refnum<class "Class Instrument Printer.lvclass"> refnum  # Library Instruments.lvlib:Class Instrument Printer.lvclass
                w193 = "" ("Address Board")
                # "Relay Board - Relay Board 16CH Acer-Micro"
                n58 = call-poly "Set (polymorphic).vi"("error in (no error)"=w198, "JSON stream"=w197) -> ("error out"=w201:errorcluster, "JSON Value out"=w199:refnum<class "JSON Value.lvclass">)  [unwired: 7 in, 1 out]
                n59 = call "JSON to Variant.vi"("error in (no error)"=w201, "Variant (Data Type)"=w193, "JSON Value"=w199) -> ("error out"=w200:errorcluster, "Variant out"=w202:variant)  [unwired: 7 in]
                n60 = Variant To Data(error in=w200, type=w193, Variant=w202) -> (data=w188:string, error out=w194:errorcluster)
                n61 = To More Generic Class(target class=refnum<class "Class Printer (Default).lvclass"> refnum ("Library Printer.lvlib:Class Printer (Default).lvclass"), reference=refnum<class "Class Printer_CAB.lvclass"> refnum ("Library Printer.lvlib:Class Printer_CAB.lvclass")) -> (generic class reference=w196:refnum<class "Class Printer (Default).lvclass">)
                n62 = Bundle By Name(cluster=T8 {"Device_Printer"="", "File To print"=path "", "Path Picture"=path "", "Library Printer"=refnum} ("Parameter"), "Library Printer"=w196, "Device_Printer"=w188) -> (w195:T8)
                n63 = To More Generic Class(target class=refnum<class "Class Instrument (Default).lvclass"> refnum ("Library Instruments.lvlib:Class Instrument (Default).lvclass"), reference=w191) -> (generic class reference=w204:refnum<class "Class Instrument (Default).lvclass">)
                n64 = To Variant(anything=w195) -> (Variant=w203:variant)
              }
              frame "Class Printer_TSC.lvclass" {
                (unwired) refnum<class "Class Printer_TSC.lvclass"> refnum  # Library Instrument & Equipement.lvlib:Library Printer.lvlib:Class Printer_TSC.lvclass
                w206 = refnum<class "Class Printer_TSC.lvclass"> refnum  # Library Printer.lvlib:Class Printer_TSC.lvclass
                w209 = refnum<class "Class Instrument Printer.lvclass"> refnum  # Library Instruments.lvlib:Class Instrument Printer.lvclass
                w211 = "" ("Address Board")
                # "Relay Board - Relay Board 16CH Acer-Micro"
                n65 = call-poly "Set (polymorphic).vi"("error in (no error)"=w216, "JSON stream"=w215) -> ("error out"=w219:errorcluster, "JSON Value out"=w217:refnum<class "JSON Value.lvclass">)  [unwired: 7 in, 1 out]
                n66 = call "JSON to Variant.vi"("error in (no error)"=w219, "Variant (Data Type)"=w211, "JSON Value"=w217) -> ("error out"=w218:errorcluster, "Variant out"=w220:variant)  [unwired: 7 in]
                n67 = Variant To Data(error in=w218, type=w211, Variant=w220) -> (data=w207:string, error out=w212:errorcluster)
                n68 = To More Generic Class(target class=refnum<class "Class Printer (Default).lvclass"> refnum ("Library Printer.lvlib:Class Printer (Default).lvclass"), reference=w206) -> (generic class reference=w214:refnum<class "Class Printer (Default).lvclass">)
                n69 = Bundle By Name(cluster=T8 {"Device_Printer"="", "File To print"=path "", "Path Picture"=path "", "Library Printer"=refnum} ("Parameter"), "Library Printer"=w214, "Device_Printer"=w207) -> (w213:T8)
                n70 = To More Generic Class(target class=refnum<class "Class Instrument (Default).lvclass"> refnum ("Library Instruments.lvlib:Class Instrument (Default).lvclass"), reference=w209) -> (generic class reference=w222:refnum<class "Class Instrument (Default).lvclass">)
                n71 = To Variant(anything=w213) -> (Variant=w221:variant)
              }
              frame "------------- Shilding Box-----------------------" {
                # "N/A"
              }
              frame "Class Shielding_ Box JC-PB3044.lvclass" {
                w228 = refnum<class "Class Shielding_ Box (Default).lvclass"> refnum  # Library Shielding box.lvlib:Class Shielding_ Box (Default).lvclass
                w227 = refnum<class "Class Shielding_ Box JC-PB3044.lvclass"> refnum  # Library Shielding box.lvlib:Class Shielding_ Box JC-PB3044.lvclass
                w230 = "" ("Address Board")
                # "Relay Board - Relay Board 16CH Acer-Micro"
                n72 = call-poly "Set (polymorphic).vi"("error in (no error)"=w235, "JSON stream"=w234) -> ("error out"=w238:errorcluster, "JSON Value out"=w236:refnum<class "JSON Value.lvclass">)  [unwired: 7 in, 1 out]
                n73 = call "JSON to Variant.vi"("error in (no error)"=w238, "Variant (Data Type)"=w230, "JSON Value"=w236) -> ("error out"=w237:errorcluster, "Variant out"=w239:variant)  [unwired: 7 in]
                n74 = Variant To Data(error in=w237, type=w230, Variant=w239) -> (data=w229:string, error out=w231:errorcluster)
                n75 = To More Generic Class(target class=w228, reference=w227) -> (generic class reference=w233:refnum<class "Class Shielding_ Box (Default).lvclass">)
                n76 = Bundle By Name(cluster=T9 {"Device @"="", "Class Shielding_ Box"=refnum} ("Parameter"), "Class Shielding_ Box"=w233, "Device @"=w229) -> (w232:T9)
                n77 = To More Generic Class(target class=refnum<class "Class Instrument (Default).lvclass"> refnum ("Library Instruments.lvlib:Class Instrument (Default).lvclass"), reference=refnum<class "Class Instrument Schielding_Box.lvclass"> refnum ("Library Instruments.lvlib:Class Instrument Schielding_Box.lvclass")) -> (generic class reference=w241:refnum<class "Class Instrument (Default).lvclass">)
                n78 = To Variant(anything=w232) -> (Variant=w240:variant)
              }
              frame "------------Spectrum Analyser--------------------" {
                # "N/A"
              }
              frame "Class Spectrum_Analyser RS306B.lvclass" {
                w247 = refnum<class "Class Spectrum_Analyser RS306B.lvclass"> refnum  # Library Spectrum Analyser.lvlib:Class Spectrum_Analyser RS306B.lvclass
                w256 = "" ("Address Board")
                # "Spectrum Analyser - RSA306B"
                n79 = call-poly "Set (polymorphic).vi"("error in (no error)"=w252, "JSON stream"=w253) -> ("error out"=w260:errorcluster, "JSON Value out"=w258:refnum<class "JSON Value.lvclass">)  [unwired: 7 in, 1 out]
                n80 = call "JSON to Variant.vi"("error in (no error)"=w260, "Variant (Data Type)"=w256, "JSON Value"=w258) -> ("error out"=w259:errorcluster, "Variant out"=w261:variant)  [unwired: 7 in]
                n81 = Variant To Data(error in=w259, type=w256, Variant=w261) -> (data=w255:string, error out=w251:errorcluster)
                n82 = To More Generic Class(target class=refnum<class "Class Spectrum Analyser (Default).lvclass"> refnum ("Library Spectrum Analyser.lvlib:Class Spectrum Analyser (Default).lvclass"), reference=w247) -> (generic class reference=w250:refnum<class "Class Spectrum Analyser (Default).lvclass">)
                n83 = Bundle By Name(cluster=T10 {"Device @"="", "Class Spectrum Analyser"=refnum, "Center Freq (MHz)"=0.0, "Freq Span (MHz)"=0.0, "Ref Level (dBm)"=0.0, "Threshold (dBm)"=0.0, "TimeOut"=0} ("Parameter"), "Class Spectrum Analyser"=w250, "Device @"=w255) -> (w257:T10)
                n84 = To Variant(anything=w257) -> (Variant=w254:variant)
                n85 = To More Generic Class(target class=refnum<class "Class Instrument (Default).lvclass"> refnum ("Library Instruments.lvlib:Class Instrument (Default).lvclass"), reference=refnum<class "Class Instrument Spectrum_Analyser.lvclass"> refnum ("Library Instruments.lvlib:Class Instrument Spectrum_Analyser.lvclass")) -> (generic class reference=w248:refnum<class "Class Instrument (Default).lvclass">)
              }
              frame "------------LED Analyser--------------------" {
                # "N/A"
              }
              frame "Class LED Analyser FEASA_10_F.lvclass" {
                w264 = refnum<class "Class LED Analyser (Default).lvclass"> refnum  # Library LED Analyser.lvlib:Class LED Analyser (Default).lvclass
                w265 = refnum<class "Class LED Analyser FEASA_10_F.lvclass"> refnum  # Library LED Analyser.lvlib:Class LED Analyser FEASA_10_F.lvclass
                w275 = "" ("Address Board")
                # "LED Analyser - FEASA 10 F"
                n86 = call-poly "Set (polymorphic).vi"("error in (no error)"=w271, "JSON stream"=w272) -> ("error out"=w279:errorcluster, "JSON Value out"=w277:refnum<class "JSON Value.lvclass">)  [unwired: 7 in, 1 out]
                n87 = call "JSON to Variant.vi"("error in (no error)"=w279, "Variant (Data Type)"=w275, "JSON Value"=w277) -> ("error out"=w278:errorcluster, "Variant out"=w280:variant)  [unwired: 7 in]
                n88 = Variant To Data(error in=w278, type=w275, Variant=w280) -> (data=w274:string, error out=w270:errorcluster)
                n89 = To More Generic Class(target class=w264, reference=w265) -> (generic class reference=w269:refnum<class "Class LED Analyser (Default).lvclass">)
                n90 = Bundle By Name(cluster=T11 {"Device @"="", "Channel"=0, "LED Analyser"=refnum} ("Parameter"), "LED Analyser"=w269, "Device @"=w274) -> (w276:T11)
                n91 = To Variant(anything=w276) -> (Variant=w273:variant)
                n92 = To More Generic Class(target class=refnum<class "Class Instrument (Default).lvclass"> refnum ("Library Instruments.lvlib:Class Instrument (Default).lvclass"), reference=refnum<class "Class Instrument LED_Analyser.lvclass"> refnum ("Library Instruments.lvlib:Class Instrument LED_Analyser.lvclass")) -> (generic class reference=w267:refnum<class "Class Instrument (Default).lvclass">)
              }
              frame "------------Database--------------------" {
                # "N/A"
              }
              frame "Firebase AssembledProducts.lvclass" {
                w283 = T21 {"Name_BDD"="", "API_Key"="", "Bench Type"=enum."Bench Assembly"} ("Parameter")
                (unwired) Bench_Type."Bench Assembly" ("Bench Type")
                w284 = refnum<class "Firebase AssembledProducts.lvclass"> refnum  # Library FireBase.lvlib:Firebase AssembledProducts.lvclass
                w298 = refnum<class "Class Instrument Firebase Altyor.lvclass"> refnum  # Library Instruments.lvlib:Class Instrument Firebase Altyor.lvclass
                w300 = refnum<class "Class Instrument (Default).lvclass"> refnum  # Library Instruments.lvlib:Class Instrument (Default).lvclass
                n93 = call-poly "Set (polymorphic).vi"("error in (no error)"=w293, "JSON stream"=w292) -> ("error out"=w296:errorcluster, "JSON Value out"=w294:refnum<class "JSON Value.lvclass">)  [unwired: 7 in, 1 out]
                n94 = call "JSON to Variant.vi"("error in (no error)"=w296, "Variant (Data Type)"=w283, "JSON Value"=w294) -> ("error out"=w295:errorcluster, "Variant out"=w297:variant)  [unwired: 7 in]
                n95 = Variant To Data(error in=w295, type=w283, Variant=w297) -> (data=w288:T21, error out=w285:errorcluster)
                n96 = Unbundle By Name(w288) -> ("Name_BDD"=w287:string, "API_Key"=w286:string, "Bench Type"=w282:T13)
                n97 = Bundle By Name(cluster=T12 {"Name_BDD"="", "API_Key"="", "Nb_to_Read"="", "Value_to_find"="", "Field_Filter"="", "Field_Order"="", "Collection_to_find"="", "Name_Bench"="", "Bench Type"=enum."Bench PCBA", "Type Data "=enum."Data Product", "Firebase Altyor"=refnum} ("Parameter"), "Firebase Altyor"=w284, "Name_BDD"=w287, "API_Key"=w286, "Bench Type"=w282) -> (w290:T12)
                n98 = To Variant(anything=w290) -> (Variant=w289:variant)
                n99 = To More Generic Class(target class=w300, reference=w298) -> (generic class reference=w299:refnum<class "Class Instrument (Default).lvclass">)
              }
              frame "Database Altyor.lvclass" {
                w304 = T22 {"Connection Name ODBC"="", "DatabaseName"=""} ("Parameter")
                (unwired) Bench_Type."Bench Assembly" ("Bench Type")
                w318 = refnum<class "Class Instrument (Default).lvclass"> refnum  # Library Instruments.lvlib:Class Instrument (Default).lvclass
                n100 = call-poly "Set (polymorphic).vi"("error in (no error)"=w312, "JSON stream"=w311) -> ("error out"=w315:errorcluster, "JSON Value out"=w313:refnum<class "JSON Value.lvclass">)  [unwired: 7 in, 1 out]
                n101 = call "JSON to Variant.vi"("error in (no error)"=w315, "Variant (Data Type)"=w304, "JSON Value"=w313) -> ("error out"=w314:errorcluster, "Variant out"=w316:variant)  [unwired: 7 in]
                n102 = Variant To Data(error in=w314, type=w304, Variant=w316) -> (data=w308:T22, error out=w305:errorcluster)
                n103 = Unbundle By Name(w308) -> ("Connection Name ODBC"=w307:string, "DatabaseName"=w306:string)
                n104 = Bundle By Name(cluster=T14 {"Connection Name ODBC"="", "DatabaseName"="", "Condition"="", "Type Data "=enum."Data Product", "Database Altyor"=refnum} ("Parameter"), "Database Altyor"=refnum<class "Database Altyor.lvclass"> refnum ("Library Database.lvlib:Database Altyor.lvclass"), "Connection Name ODBC"=w307, "DatabaseName"=w306) -> (w310:T14)
                n105 = To Variant(anything=w310) -> (Variant=w309:variant)
                n106 = To More Generic Class(target class=w318, reference=refnum<class "Class Instrument Database Altyor.lvclass"> refnum ("Library Instruments.lvlib:Class Instrument Database Altyor.lvclass")) -> (generic class reference=w317:refnum<class "Class Instrument (Default).lvclass">)
              }
              frame "Firebase Benches.lvclass" {
                w321 = T21 {"Name_BDD"="", "API_Key"="", "Bench Type"=enum."Bench PCBA"} ("Parameter")
                w328 = refnum<class "Firebase Benches.lvclass"> refnum  # Library FireBase.lvlib:Firebase Benches.lvclass
                w339 = refnum<class "Class Instrument (Default).lvclass"> refnum  # Library Instruments.lvlib:Class Instrument (Default).lvclass
                n107 = call-poly "Set (polymorphic).vi"("error in (no error)"=w332, "JSON stream"=w319) -> ("error out"=w335:errorcluster, "JSON Value out"=w333:refnum<class "JSON Value.lvclass">)  [unwired: 7 in, 1 out]
                n108 = call "JSON to Variant.vi"("error in (no error)"=w335, "Variant (Data Type)"=w321, "JSON Value"=w333) -> ("error out"=w334:errorcluster, "Variant out"=w336:variant)  [unwired: 7 in]
                n109 = Variant To Data(error in=w334, type=w321, Variant=w336) -> (data=w327:T21, error out=w324:errorcluster)
                n110 = Unbundle By Name(w327) -> ("Name_BDD"=w326:string, "API_Key"=w325:string, "Bench Type"=w320:T13)
                n111 = case shown="\"Bench Camera\"" w320 {
                  tunnel: ["PCBA" ("Name_Bench") "CAM" ("Name_Bench")] -> w323
                  frame "Bench PCBA", Default {
                  }
                  frame "Bench Camera" {
                  }
                }
                n112 = Bundle By Name(cluster=T12 {"Name_BDD"="", "API_Key"="", "Nb_to_Read"="", "Value_to_find"="", "Field_Filter"="", "Field_Order"="", "Collection_to_find"="", "Name_Bench"="", "Bench Type"=enum."Bench PCBA", "Type Data "=enum."Data Product", "Firebase Altyor"=refnum} ("Parameter"), "Firebase Altyor"=w328, "Name_BDD"=w326, "API_Key"=w325, "Bench Type"=w320, "Name_Bench"=w323, "Value_to_find"=w323, "Collection_to_find"="Benches") -> (w330:T12)
                n113 = To Variant(anything=w330) -> (Variant=w329:variant)
                n114 = To More Generic Class(target class=w339, reference=refnum<class "Class Instrument Firebase Altyor.lvclass"> refnum ("Library Instruments.lvlib:Class Instrument Firebase Altyor.lvclass")) -> (generic class reference=w338:refnum<class "Class Instrument (Default).lvclass">)
              }
              frame "------------- UART -----------------------" {
              }
              frame "Class UART Enocean.lvclass" {
                w352 = T23 {"Address Device"="", "Baud Rate"=0, "Data Bit"=0, "stop bits (10: 1 bit)"=10, "parity (0:none)"=enum."None", "flow control (0:none)"=0, "termination char "=10, "Enable Termination"=TRUE} ("Parameter")
                w366 = refnum<class "Class Instrument (Default).lvclass"> refnum  # Library Instruments.lvlib:Class Instrument (Default).lvclass
                n115 = call-poly "Set (polymorphic).vi"("error in (no error)"=w360, "JSON stream"=w359) -> ("error out"=w363:errorcluster, "JSON Value out"=w361:refnum<class "JSON Value.lvclass">)  [unwired: 7 in, 1 out]
                n116 = call "JSON to Variant.vi"("error in (no error)"=w363, "Variant (Data Type)"=w352, "JSON Value"=w361) -> ("error out"=w362:errorcluster, "Variant out"=w364:variant)  [unwired: 7 in]
                n117 = Variant To Data(error in=w362, type=w352, Variant=w364) -> (data=w351:T23, error out=w356:errorcluster)
                n118 = Unbundle By Name(w351) -> ("Address Device"=w350:refnum<visa-resource-name>, "Baud Rate"=w349:u32, "Data Bit"=w348:u16, "stop bits (10: 1 bit)"=w347:u16, "parity (0:none)"=w346:enum16{"None", "Odd", "Even", "Mark", "Space"}, "flow control (0:none)"=w345:u16, "termination char"=w344:u8, "Enable Termination"=w343:bool)
                n119 = Bundle By Name(cluster=T15 {"Address Device"="", "Baud Rate"=0, "Data Bit"=0, "stop bits (10: 1 bit)"=0, "parity (0:none)"=enum."None", "flow control (0:none)"=0, "termination char "=0, "Enable Termination"=FALSE, "Nb Octet to Read"=0, "Class UART"=refnum} ("Parameter"), "Class UART"=refnum<class "Class UART Enocean.lvclass"> refnum ("Library UART.lvlib:Class UART Enocean.lvclass"), "Address Device"=w350, "Baud Rate"=w349, "Data Bit"=w348, "stop bits (10: 1 bit)"=w347, "parity (0:none)"=w346, "flow control (0:none)"=w345, "termination char"=w344, "Enable Termination"=w343) -> (w358:T15)
                n120 = To Variant(anything=w358) -> (Variant=w357:variant)
                n121 = To More Generic Class(target class=w366, reference=refnum<class "Class Instrument UART.lvclass"> refnum ("Library Instruments.lvlib:Class Instrument UART.lvclass")) -> (generic class reference=w365:refnum<class "Class Instrument (Default).lvclass">)
              }
              frame "Class UART Nodon.lvclass" {
                w377 = T23 {"Address Device"="", "Baud Rate"=0, "Data Bit"=0, "stop bits (10: 1 bit)"=10, "parity (0:none)"=enum."None", "flow control (0:none)"=0, "termination char "=10, "Enable Termination"=TRUE} ("Parameter")
                w390 = refnum<class "Class Instrument (Default).lvclass"> refnum  # Library Instruments.lvlib:Class Instrument (Default).lvclass
                n122 = call-poly "Set (polymorphic).vi"("error in (no error)"=w384, "JSON stream"=w383) -> ("error out"=w387:errorcluster, "JSON Value out"=w385:refnum<class "JSON Value.lvclass">)  [unwired: 7 in, 1 out]
                n123 = call "JSON to Variant.vi"("error in (no error)"=w387, "Variant (Data Type)"=w377, "JSON Value"=w385) -> ("error out"=w386:errorcluster, "Variant out"=w388:variant)  [unwired: 7 in]
                n124 = Variant To Data(error in=w386, type=w377, Variant=w388) -> (data=w376:T23, error out=w380:errorcluster)
                n125 = Unbundle By Name(w376) -> ("Address Device"=w375:refnum<visa-resource-name>, "Baud Rate"=w374:u32, "Data Bit"=w373:u16, "stop bits (10: 1 bit)"=w372:u16, "parity (0:none)"=w371:enum16{"None", "Odd", "Even", "Mark", "Space"}, "flow control (0:none)"=w370:u16, "termination char"=w369:u8, "Enable Termination"=w368:bool)
                n126 = Bundle By Name(cluster=T15 {"Address Device"="", "Baud Rate"=0, "Data Bit"=0, "stop bits (10: 1 bit)"=0, "parity (0:none)"=enum."None", "flow control (0:none)"=0, "termination char "=0, "Enable Termination"=FALSE, "Nb Octet to Read"=0, "Class UART"=refnum} ("Parameter"), "Class UART"=refnum<class "Class UART Nodon.lvclass"> refnum ("Library UART.lvlib:Class UART Nodon.lvclass"), "Address Device"=w375, "Baud Rate"=w374, "Data Bit"=w373, "stop bits (10: 1 bit)"=w372, "parity (0:none)"=w371, "flow control (0:none)"=w370, "termination char"=w369, "Enable Termination"=w368) -> (w382:T15)
                n127 = To Variant(anything=w382) -> (Variant=w381:variant)
                n128 = To More Generic Class(target class=w390, reference=refnum<class "Class Instrument UART.lvclass"> refnum ("Library Instruments.lvlib:Class Instrument UART.lvclass")) -> (generic class reference=w389:refnum<class "Class Instrument (Default).lvclass">)
              }
              frame "Class UART P2056.lvclass" {
                w401 = T23 {"Address Device"="", "Baud Rate"=0, "Data Bit"=0, "stop bits (10: 1 bit)"=10, "parity (0:none)"=enum."None", "flow control (0:none)"=0, "termination char "=10, "Enable Termination"=TRUE} ("Parameter")
                w414 = refnum<class "Class Instrument (Default).lvclass"> refnum  # Library Instruments.lvlib:Class Instrument (Default).lvclass
                n129 = call-poly "Set (polymorphic).vi"("error in (no error)"=w408, "JSON stream"=w407) -> ("error out"=w411:errorcluster, "JSON Value out"=w409:refnum<class "JSON Value.lvclass">)  [unwired: 7 in, 1 out]
                n130 = call "JSON to Variant.vi"("error in (no error)"=w411, "Variant (Data Type)"=w401, "JSON Value"=w409) -> ("error out"=w410:errorcluster, "Variant out"=w412:variant)  [unwired: 7 in]
                n131 = Variant To Data(error in=w410, type=w401, Variant=w412) -> (data=w400:T23, error out=w404:errorcluster)
                n132 = Unbundle By Name(w400) -> ("Address Device"=w399:refnum<visa-resource-name>, "Baud Rate"=w398:u32, "Data Bit"=w397:u16, "stop bits (10: 1 bit)"=w396:u16, "parity (0:none)"=w395:enum16{"None", "Odd", "Even", "Mark", "Space"}, "flow control (0:none)"=w394:u16, "termination char"=w393:u8, "Enable Termination"=w392:bool)
                n133 = Bundle By Name(cluster=T15 {"Address Device"="", "Baud Rate"=0, "Data Bit"=0, "stop bits (10: 1 bit)"=0, "parity (0:none)"=enum."None", "flow control (0:none)"=0, "termination char "=0, "Enable Termination"=FALSE, "Nb Octet to Read"=0, "Class UART"=refnum} ("Parameter"), "Class UART"=refnum<class "Class UART P2056.lvclass"> refnum ("Library UART.lvlib:Class UART P2056.lvclass"), "Address Device"=w399, "Baud Rate"=w398, "Data Bit"=w397, "stop bits (10: 1 bit)"=w396, "parity (0:none)"=w395, "flow control (0:none)"=w394, "termination char"=w393, "Enable Termination"=w392) -> (w406:T15)
                n134 = To Variant(anything=w406) -> (Variant=w405:variant)
                n135 = To More Generic Class(target class=w414, reference=refnum<class "Class Instrument UART.lvclass"> refnum ("Library Instruments.lvlib:Class Instrument UART.lvclass")) -> (generic class reference=w413:refnum<class "Class Instrument (Default).lvclass">)
              }
              frame "Class UART Zigbee.lvclass" {
                w425 = T23 {"Address Device"="", "Baud Rate"=0, "Data Bit"=0, "stop bits (10: 1 bit)"=10, "parity (0:none)"=enum."None", "flow control (0:none)"=0, "termination char "=10, "Enable Termination"=TRUE} ("Parameter")
                w438 = refnum<class "Class Instrument (Default).lvclass"> refnum  # Library Instruments.lvlib:Class Instrument (Default).lvclass
                n136 = call-poly "Set (polymorphic).vi"("error in (no error)"=w432, "JSON stream"=w431) -> ("error out"=w435:errorcluster, "JSON Value out"=w433:refnum<class "JSON Value.lvclass">)  [unwired: 7 in, 1 out]
                n137 = call "JSON to Variant.vi"("error in (no error)"=w435, "Variant (Data Type)"=w425, "JSON Value"=w433) -> ("error out"=w434:errorcluster, "Variant out"=w436:variant)  [unwired: 7 in]
                n138 = Variant To Data(error in=w434, type=w425, Variant=w436) -> (data=w424:T23, error out=w428:errorcluster)
                n139 = Unbundle By Name(w424) -> ("Address Device"=w423:refnum<visa-resource-name>, "Baud Rate"=w422:u32, "Data Bit"=w421:u16, "stop bits (10: 1 bit)"=w420:u16, "parity (0:none)"=w419:enum16{"None", "Odd", "Even", "Mark", "Space"}, "flow control (0:none)"=w418:u16, "termination char"=w417:u8, "Enable Termination"=w416:bool)
                n140 = Bundle By Name(cluster=T15 {"Address Device"="", "Baud Rate"=0, "Data Bit"=0, "stop bits (10: 1 bit)"=0, "parity (0:none)"=enum."None", "flow control (0:none)"=0, "termination char "=0, "Enable Termination"=FALSE, "Nb Octet to Read"=0, "Class UART"=refnum} ("Parameter"), "Class UART"=refnum<class "Class UART Zigbee.lvclass"> refnum ("Library UART.lvlib:Class UART Zigbee.lvclass"), "Address Device"=w423, "Baud Rate"=w422, "Data Bit"=w421, "stop bits (10: 1 bit)"=w420, "parity (0:none)"=w419, "flow control (0:none)"=w418, "termination char"=w417, "Enable Termination"=w416) -> (w430:T15)
                n141 = To Variant(anything=w430) -> (Variant=w429:variant)
                n142 = To More Generic Class(target class=w438, reference=refnum<class "Class Instrument UART.lvclass"> refnum ("Library Instruments.lvlib:Class Instrument UART.lvclass")) -> (generic class reference=w437:refnum<class "Class Instrument (Default).lvclass">)
              }
              frame "----------Pattern_Matching-----------------" {
              }
              frame "Class Camera IV3-500CA.lvclass" {
                w441 = cluster{"Device_Addr":string, "Port":string} {"Device_Addr"="", "Port"=""} ("Parameter")
                w443 = refnum<class "Class Instrument Patterm_Matching.lvclass"> refnum  # Library Instruments.lvlib:Class Instrument Patterm_Matching.lvclass
                w444 = refnum<class "Class Camera IV3-500CA.lvclass"> refnum  # Library Camera.lvlib:Class Camera IV3-500CA.lvclass
                w458 = refnum<class "Class Instrument (Default).lvclass"> refnum  # Library Instruments.lvlib:Class Instrument (Default).lvclass
                n143 = call-poly "Set (polymorphic).vi"("error in (no error)"=w452, "JSON stream"=w451) -> ("error out"=w455:errorcluster, "JSON Value out"=w453:refnum<class "JSON Value.lvclass">)  [unwired: 7 in, 1 out]
                n144 = call "JSON to Variant.vi"("error in (no error)"=w455, "Variant (Data Type)"=w441, "JSON Value"=w453) -> ("error out"=w454:errorcluster, "Variant out"=w456:variant)  [unwired: 7 in]
                n145 = Variant To Data(error in=w454, type=w441, Variant=w456) -> (data=w447:cluster{"Device_Addr":string, "Port":string}, error out=w448:errorcluster)
                n146 = Unbundle By Name(w447) -> ("Device_Addr"=w446:string, "Port"=w445:string)
                n147 = Bundle By Name(cluster=T16 {"Device_Addr"="", "Port"="", "Number Prog"="", "Test Number"=0, "Timeout"=0, "Library Pattern Matching"=refnum} ("Parameter"), "Library Pattern Matching"=w444, "Device_Addr"=w446, "Port"=w445, "Timeout"=u16 2000) -> (w450:T16)
                n148 = To Variant(anything=w450) -> (Variant=w449:variant)
                n149 = To More Generic Class(target class=w458, reference=w443) -> (generic class reference=w457:refnum<class "Class Instrument (Default).lvclass">)
              }
              frame "--------------------Balance---------------" {
              }
              frame "Class Balance_Adam_GBK.lvclass" {
                w464 = cluster{"Address Device":string, "Timeout":u32} {"Address Device"="", "Timeout"=0} ("Parameter")
                # "Balance - Adam_GBK"
                n150 = call-poly "Set (polymorphic).vi"("error in (no error)"=w472, "JSON stream"=w473) -> ("error out"=w478:errorcluster, "JSON Value out"=w476:refnum<class "JSON Value.lvclass">)  [unwired: 7 in, 1 out]
                n151 = call "JSON to Variant.vi"("error in (no error)"=w478, "Variant (Data Type)"=w464, "JSON Value"=w476) -> ("error out"=w477:errorcluster, "Variant out"=w479:variant)  [unwired: 7 in]
                n152 = Variant To Data(error in=w477, type=w464, Variant=w479) -> (data=w463:cluster{"Address Device":string, "Timeout":u32}, error out=w471:errorcluster)
                n153 = Unbundle By Name(w463) -> ("Address Device"=w462:string, "Timeout"=w461:u32)
                n154 = To More Generic Class(target class=refnum<class "Class Balance (Default).lvclass"> refnum ("Library Balance.lvlib:Class Balance (Default).lvclass"), reference=refnum<class "Class Balance_Adam_GBK.lvclass"> refnum ("Library Balance.lvlib:Class Balance_Adam_GBK.lvclass")) -> (generic class reference=w470:refnum<class "Class Balance (Default).lvclass">)
                n155 = Bundle By Name(cluster=T17 {"Device @"="", "Timeout"=0, "Class Balance"=refnum} ("Parameter"), "Class Balance"=w470, "Device @"=w462, "Timeout"=w461) -> (w475:T17)
                n156 = To Variant(anything=w475) -> (Variant=w474:variant)
                n157 = To More Generic Class(target class=refnum<class "Class Instrument (Default).lvclass"> refnum ("Library Instruments.lvlib:Class Instrument (Default).lvclass"), reference=refnum<class "Class Instrument Balance.lvclass"> refnum ("Library Instruments.lvlib:Class Instrument Balance.lvclass")) -> (generic class reference=w468:refnum<class "Class Instrument (Default).lvclass">)
              }
              frame "-------------Log File----------" {
              }
              frame "Class Log_File Altyor.lvclass" {
                w486 = refnum<class "Class Instrument Log_File.lvclass"> refnum  # Library Instruments.lvlib:Class Instrument Log_File.lvclass
                w487 = cluster{"Path Historic":path} {"Path Historic"=path ""} ("Parameter")
                w498 = refnum<class "Class Instrument (Default).lvclass"> refnum  # Library Instruments.lvlib:Class Instrument (Default).lvclass
                n158 = call-poly "Set (polymorphic).vi"("error in (no error)"=w492, "JSON stream"=w481) -> ("error out"=w495:errorcluster, "JSON Value out"=w493:refnum<class "JSON Value.lvclass">)  [unwired: 7 in, 1 out]
                n159 = call "JSON to Variant.vi"("error in (no error)"=w495, "Variant (Data Type)"=w487, "JSON Value"=w493) -> ("error out"=w494:errorcluster, "Variant out"=w496:variant)  [unwired: 7 in]
                n160 = Variant To Data(error in=w494, type=w487, Variant=w496) -> (data=w488:cluster{"Path Historic":path}, error out=w489:errorcluster)
                n161 = Unbundle By Name(w488) -> ("Path Historic"=w484:path)
                n162 = Bundle By Name(cluster=T18 {"Path_Log_File"=path "", "Delimit"="", "File For Save"=refnum, "Event Error"=refnum, "Class Log_File"=refnum} ("Parameter"), "Class Log_File"=refnum<class "Class Log_File Altyor.lvclass"> refnum ("Library Log_File.lvlib:Class Log_File Altyor.lvclass"), "Path_Log_File"=w484, "Delimit"=";") -> (w491:T18)
                n163 = To Variant(anything=w491) -> (Variant=w490:variant)
                n164 = To More Generic Class(target class=w498, reference=w486) -> (generic class reference=w497:refnum<class "Class Instrument (Default).lvclass">)
              }
              frame Default {
                (unwired) refnum<class "Class Instrument (Default).lvclass"> refnum ("Library Instruments.lvlib:Class Instrument (Default).lvclass")
                # "Error, class not found"
              }
            }
            n165 = call-poly "Set (polymorphic).vi"("error in (no error)"=w36, "Variant"=w27) -> ("error out"=w37:errorcluster, "JSON Value out"=w33:refnum<class "JSON Value.lvclass">)  [unwired: 8 in]
            n166 = call "Get as JSON string.vi"("error in (no error)"=w37, "JSON Value in"=w33) -> ("error out"=w29:errorcluster, "<JSON>"=w32:string)  [unwired: 8 in]
            n167 = property class="Class Instrument (Default).lvcl"(reference=w35, error in=w29, "Property:Parameter_Json"=w32, "Property:Instrument_name "=w31) -> (reference out=w34:refnum<class "Class Instrument (Default).lvclass">, error out=w28:errorcluster)
          }
          frame "Save Insrt obj" {
          }
          frame "Get Instr obj" {
            n168 = for {
              tunnel: w505 -> [w510] mode=indexing
              tunnel: w504 -> [w508]
              tunnel: [w507] -> w503
              tunnel: [w506] -> _
              stop <- w506 stop-if-true
              n169 = Unbundle By Name(w510) -> ("Instrument"=w507:refnum<class "Class Instrument (Default).lvclass">, "Name"=w509:string)
              n170 = Equal?(x=w509, y=w508) -> (x = y?=w506:bool)
            }
          }
          frame "Modify Insrt obj" {
            n171 = for {
              tunnel: w516 -> [w526] mode=indexing
              tunnel: w520 -> [w530]
              tunnel: [w529] -> w519
              tunnel: [w528] -> w512
              tunnel: [w527] -> w517
              tunnel: [w526] -> w515
              i -> [w527]
              stop <- w528 stop-if-true
              n172 = Unbundle By Name(w526) -> ("Instrument"=w529:refnum<class "Class Instrument (Default).lvclass">, "Name"=w531:string)
              n173 = Equal?(x=w531, y=w530) -> (x = y?=w528:bool)
            }
            n174 = Bundle By Name(cluster=w515, "Instrument"="Familly class IN") -> (w513:T24)
            n175 = case shown="Faux" w512 {
              tunnel: [w521 w524] -> w511
              tunnel: w517 -> [_ w525]
              tunnel: w516 -> [w521 w523]
              tunnel: w513 -> [_ w522]
              frame False {
              }
              frame True {
                n176 = Replace Array Subset(array=w523, new element=w522, index=w525) -> (w524:T1)
              }
            }
          }
          frame "List Instr" {
            "Instruments 2" <- w532
          }
        }
      }
    }
    frame Error {
    }
  }
  "error out" <- w6
  "Familly class Out" <- w2
